vi "TCC.vi"() -> (2 "State out":string="Data: Load Thermal Calibration")   [LabVIEW 2020]
uses:
  DataCluster_TCAL.ctl
  <vilib>/vision/Image Controls.llb/IMAQ Image.ctl
  DataCluster.ctl
  <vilib>/userdefined/High Color/IMAQdx.ctl
  <vilib>/Utility/xml.llb/Write to XML File(string).vi
panel:
  out "Pict Ring":i32(ring)
  in  "Done":bool
  out "Step":string="Step: 4\n\nCalculate temperature!"
  in  "Fixpoint Radius":i32=20 min=3 max=20
  in  "Cluster":T1 {"PCR Size" items=["384 (24x16)", "96 (12x8)"]; "Points"."Top Left"."Y" format="%.2f"; "Points"."Top Left"."X" format="%.2f"; "Points"."Top Right"."Y" format="%.2f"; "Points"."Top Right"."X" format="%.2f"; "Points"."Bottom Left"."Y" format="%.2f"; "Points"."Bottom Left"."X" format="%.2f"; "Points"."Bottom Right"."Y" format="%.2f"; "Points"."Bottom Right"."X" format="%.2f"; "Points"."Fixpoint"."Y" format="%.2f"; "Points"."Fixpoint"."X" format="%.2f"}
  in  "Display Mapping":u32(ring)=10 items=["Default"=10, "Most Significant Bits"=11, "Full Dynamic"=12, "Downshift"=13, "Given Range"=14, "90% Dynamic"=15, "Given Percent Range"=16]
  in  "Image":u32(slide) scale=0.0..242.0
  in  "Help":bool
  out "Tutorial":string="Step: 4\n\nCalculate temperature!"
  in  "Show All Points":bool
  in  "Well Radius":u32=50 min=1 max=100
  in  "PCR Size":u16(ring) items=["384 (24x16)", "96 (12x8)"]
  out "Points":T3[](array[typedef])=[{"X"=103.0, "Y"=94.0}, {"X"=158.04349, "Y"=93.521736}, {"X"=213.08696, "Y"=93.04348}, {"X"=268.13043, "Y"=92.565216}, {"X"=323.17392, "Y"=92.08696}, {"X"=378.2174, "Y"=91.608696}, {"X"=433.26086, "Y"=91.13043}, {"X"=488.30435, "Y"=90.652176}, {"X"=543.34784, "Y"=90.17391}, {"X"=598.39136, "Y"=89.69565}, {"X"=653.4348, "Y"=89.21739}, {"X"=708.4783, "Y"=88.73913}, {"X"=763.5217, "Y"=88.26087}, {"X"=818.56525, "Y"=87.78261}, {"X"=873.6087, "Y"=87.30435}, {"X"=928.6522, "Y"=86.82609}, {"X"=983.6957, "Y"=86.347824}, {"X"=1038.7391, "Y"=85.86957}, {"X"=1093.7827, "Y"=85.391304}, {"X"=1148.8262, "Y"=84.91304}, {"X"=1203.8696, "Y"=84.434784}, {"X"=1258.9131, "Y"=83.95652}, {"X"=1313.9565, "Y"=83.478264}, {"X"=1369.0, "Y"=83.0}, {"X"=103.46667, "Y"=149.06667}, {"X"=158.51015, "Y"=148.58841}, {"X"=213.55362, "Y"=148.11014}, {"X"=268.5971, "Y"=147.63188}, {"X"=323.6406, "Y"=147.15363}, {"X"=378.68408, "Y"=146.67535}, {"X"=433.72754, "Y"=146.1971}, {"X"=488.77103, "Y"=145.71884}, {"X"=543.8145, "Y"=145.24057}, {"X"=598.858, "Y"=144.76231}, {"X"=653.9015, "Y"=144.28406}, {"X"=708.94495, "Y"=143.8058}, {"X"=763.9884, "Y"=143.32753}, {"X"=819.0319, "Y"=142.84927}, {"X"=874.0754, "Y"=142.37102}, {"X"=929.1189, "Y"=141.89276}, {"X"=984.16235, "Y"=141.41449}, {"X"=1039.2058, "Y"=140.93623}, {"X"=1094.2493, "Y"=140.45798}, {"X"=1149.2928, "Y"=139.9797}, {"X"=1204.3363, "Y"=139.50145}, {"X"=1259.3798, "Y"=139.0232}, {"X"=1314.4232, "Y"=138.54492}, {"X"=1369.4667, "Y"=138.06667}, {"X"=103.933334, "Y"=204.13333}, {"X"=158.9768, "Y"=203.65506}, {"X"=214.0203, "Y"=203.17682}, {"X"=269.06375, "Y"=202.69855}, {"X"=324.10724, "Y"=202.22029}, {"X"=379.15073, "Y"=201.74203}, {"X"=434.19418, "Y"=201.26376}, {"X"=489.23767, "Y"=200.7855}, {"X"=544.2812, "Y"=200.30725}, {"X"=599.32465, "Y"=199.82898}, {"X"=654.36816, "Y"=199.35072}, {"X"=709.4116, "Y"=198.87247}, {"X"=764.4551, "Y"=198.3942}, {"X"=819.4986, "Y"=197.91594}, {"X"=874.54205, "Y"=197.43768}, {"X"=929.5856, "Y"=196.95941}, {"X"=984.629, "Y"=196.48116}, {"X"=1039.6725, "Y"=196.0029}, {"X"=1094.716, "Y"=195.52463}, {"X"=1149.7595, "Y"=195.04637}, {"X"=1204.803, "Y"=194.56812}, {"X"=1259.8464, "Y"=194.08984}, {"X"=1314.8899, "Y"=193.6116}, {"X"=1369.9333, "Y"=193.13333}, {"X"=104.4, "Y"=259.2}, {"X"=159.44348, "Y"=258.72174}, {"X"=214.48695, "Y"=258.24347}, {"X"=269.53043, "Y"=257.7652}, {"X"=324.5739, "Y"=257.28696}, {"X"=379.6174, "Y"=256.8087}, {"X"=434.66086, "Y"=256.33044}, {"X"=489.70435, "Y"=255.85217}, {"X"=544.74786, "Y"=255.37392}, {"X"=599.7913, "Y"=254.89565}, {"X"=654.83484, "Y"=254.41739}, {"X"=709.8783, "Y"=253.93913}, {"X"=764.92175, "Y"=253.46086}, {"X"=819.9653, "Y"=252.9826}, {"X"=875.0087, "Y"=252.50435}, {"X"=930.05225, "Y"=252.02608}, {"X"=985.0957, "Y"=251.54782}, {"X"=1040.1392, "Y"=251.06956}, {"X"=1095.1826, "Y"=250.59131}, {"X"=1150.2262, "Y"=250.11304}, {"X"=1205.2697, "Y"=249.63478}, {"X"=1260.3131, "Y"=249.15652}, {"X"=1315.3566, "Y"=248.67825}, {"X"=1370.4, "Y"=248.2}, {"X"=104.86667, "Y"=314.26666}, {"X"=159.91014, "Y"=313.7884}, {"X"=214.95363, "Y"=313.31012}, {"X"=269.9971, "Y"=312.83188}, {"X"=325.0406, "Y"=312.35364}, {"X"=380.08408, "Y"=311.87537}, {"X"=435.12753, "Y"=311.3971}, {"X"=490.17102, "Y"=310.91882}, {"X"=545.2145, "Y"=310.44058}, {"X"=600.258, "Y"=309.9623}, {"X"=655.30145, "Y"=309.48407}, {"X"=710.3449, "Y"=309.0058}, {"X"=765.38837, "Y"=308.52753}, {"X"=820.4319, "Y"=308.04926}, {"X"=875.47534, "Y"=307.571}, {"X"=930.51886, "Y"=307.09274}, {"X"=985.5623, "Y"=306.6145}, {"X"=1040.6058, "Y"=306.13623}, {"X"=1095.6493, "Y"=305.65796}, {"X"=1150.6929, "Y"=305.1797}, {"X"=1205.7363, "Y"=304.70145}, {"X"=1260.7798, "Y"=304.2232}, {"X"=1315.8232, "Y"=303.74493}, {"X"=1370.8667, "Y"=303.26666}, {"X"=105.333336, "Y"=369.3333}, {"X"=160.37682, "Y"=368.85504}, {"X"=215.42029, "Y"=368.3768}, {"X"=270.46378, "Y"=367.89853}, {"X"=325.50726, "Y"=367.42026}, {"X"=380.55075, "Y"=366.94202}, {"X"=435.5942, "Y"=366.46375}, {"X"=490.6377, "Y"=365.98547}, {"X"=545.68115, "Y"=365.50723}, {"X"=600.7247, "Y"=365.02896}, {"X"=655.7681, "Y"=364.5507}, {"X"=710.8116, "Y"=364.07245}, {"X"=765.85504, "Y"=363.59418}, {"X"=820.89856, "Y"=363.11594}, {"X"=875.942, "Y"=362.63766}, {"X"=930.98553, "Y"=362.1594}, {"X"=986.029, "Y"=361.68115}, {"X"=1041.0725, "Y"=361.20288}, {"X"=1096.116, "Y"=360.7246}, {"X"=1151.1595, "Y"=360.24637}, {"X"=1206.203, "Y"=359.7681}, {"X"=1261.2465, "Y"=359.28983}, {"X"=1316.2899, "Y"=358.81158}, {"X"=1371.3334, "Y"=358.3333}, {"X"=105.8, "Y"=424.4}, {"X"=160.84348, "Y"=423.92172}, {"X"=215.88696, "Y"=423.44348}, {"X"=270.93042, "Y"=422.9652}, {"X"=325.9739, "Y"=422.48694}, {"X"=381.0174, "Y"=422.0087}, {"X"=436.06085, "Y"=421.53043}, {"X"=491.10434, "Y"=421.05215}, {"X"=546.1478, "Y"=420.5739}, {"X"=601.19135, "Y"=420.09564}, {"X"=656.2348, "Y"=419.61737}, {"X"=711.27826, "Y"=419.13913}, {"X"=766.3217, "Y"=418.66086}, {"X"=821.36523, "Y"=418.18262}, {"X"=876.4087, "Y"=417.70435}, {"X"=931.4522, "Y"=417.22607}, {"X"=986.49567, "Y"=416.74783}, {"X"=1041.5392, "Y"=416.26956}, {"X"=1096.5826, "Y"=415.7913}, {"X"=1151.6262, "Y"=415.31305}, {"X"=1206.6697, "Y"=414.83478}, {"X"=1261.7131, "Y"=414.3565}, {"X"=1316.7566, "Y"=413.87827}, {"X"=1371.8, "Y"=413.4}, {"X"=106.26667, "Y"=479.46667}, {"X"=161.31015, "Y"=478.9884}, {"X"=216.35362, "Y"=478.51016}, {"X"=271.3971, "Y"=478.0319}, {"X"=326.44058, "Y"=477.55362}, {"X"=381.48407, "Y"=477.07538}, {"X"=436.52753, "Y"=476.5971}, {"X"=491.571, "Y"=476.11884}, {"X"=546.6145, "Y"=475.6406}, {"X"=601.658, "Y"=475.16232}, {"X"=656.7015, "Y"=474.68405}, {"X"=711.74493, "Y"=474.2058}, {"X"=766.7884, "Y"=473.72754}, {"X"=821.8319, "Y"=473.2493}, {"X"=876.87537, "Y"=472.77103}, {"X"=931.9189, "Y"=472.29276}, {"X"=986.96234, "Y"=471.8145}, {"X"=1042.0059, "Y"=471.33624}, {"X"=1097.0493, "Y"=470.85797}, {"X"=1152.0929, "Y"=470.37973}, {"X"=1207.1364, "Y"=469.90146}, {"X"=1262.1798, "Y"=469.4232}, {"X"=1317.2233, "Y"=468.94495}, {"X"=1372.2667, "Y"=468.46667}, {"X"=106.73333, "Y"=534.5333}, {"X"=161.77681, "Y"=534.05505}, {"X"=216.8203, "Y"=533.5768}, {"X"=271.86377, "Y"=533.0985}, {"X"=326.90726, "Y"=532.62024}, {"X"=381.95074, "Y"=532.142}, {"X"=436.9942, "Y"=531.66376}, {"X"=492.0377, "Y"=531.1855}, {"X"=547.0812, "Y"=530.7073}, {"X"=602.12463, "Y"=530.229}, {"X"=657.16815, "Y"=529.75073}, {"X"=712.2116, "Y"=529.27246}, {"X"=767.25507, "Y"=528.7942}, {"X"=822.2986, "Y"=528.3159}, {"X"=877.34204, "Y"=527.83765}, {"X"=932.38556, "Y"=527.3594}, {"X"=987.429, "Y"=526.88116}, {"X"=1042.4724, "Y"=526.4029}, {"X"=1097.516, "Y"=525.9246}, {"X"=1152.5594, "Y"=525.4464}, {"X"=1207.6029, "Y"=524.96814}, {"X"=1262.6464, "Y"=524.48987}, {"X"=1317.6898, "Y"=524.0116}, {"X"=1372.7333, "Y"=523.5333}, {"X"=107.2, "Y"=589.6}, {"X"=162.24348, "Y"=589.1217}, {"X"=217.28696, "Y"=588.64343}, {"X"=272.33044, "Y"=588.16516}, {"X"=327.37393, "Y"=587.6869}, {"X"=382.41742, "Y"=587.2087}, {"X"=437.46088, "Y"=586.7304}, {"X"=492.50436, "Y"=586.25214}, {"X"=547.54785, "Y"=585.7739}, {"X"=602.5913, "Y"=585.29565}, {"X"=657.6348, "Y"=584.8174}, {"X"=712.6783, "Y"=584.3391}, {"X"=767.72174, "Y"=583.86084}, {"X"=822.76526, "Y"=583.38257}, {"X"=877.8087, "Y"=582.9043}, {"X"=932.85223, "Y"=582.426}, {"X"=987.8957, "Y"=581.9478}, {"X"=1042.9391, "Y"=581.46954}, {"X"=1097.9827, "Y"=580.9913}, {"X"=1153.0261, "Y"=580.51306}, {"X"=1208.0696, "Y"=580.0348}, {"X"=1263.113, "Y"=579.5565}, {"X"=1318.1565, "Y"=579.07825}, {"X"=1373.2, "Y"=578.6}, {"X"=107.666664, "Y"=644.6666}, {"X"=162.71014, "Y"=644.18835}, {"X"=217.75363, "Y"=643.7101}, {"X"=272.7971, "Y"=643.2319}, {"X"=327.84058, "Y"=642.7536}, {"X"=382.88406, "Y"=642.2753}, {"X"=437.92752, "Y"=641.79706}, {"X"=492.971, "Y"=641.3188}, {"X"=548.0145, "Y"=640.8405}, {"X"=603.058, "Y"=640.3623}, {"X"=658.1015, "Y"=639.88403}, {"X"=713.14496, "Y"=639.40576}, {"X"=768.1884, "Y"=638.9275}, {"X"=823.23193, "Y"=638.4492}, {"X"=878.2754, "Y"=637.97095}, {"X"=933.3189, "Y"=637.49274}, {"X"=988.36237, "Y"=637.01447}, {"X"=1043.4058, "Y"=636.5362}, {"X"=1098.4493, "Y"=636.0579}, {"X"=1153.4928, "Y"=635.57965}, {"X"=1208.5363, "Y"=635.1014}, {"X"=1263.5797, "Y"=634.62317}, {"X"=1318.6232, "Y"=634.1449}, {"X"=1373.6666, "Y"=633.6666}, {"X"=108.13333, "Y"=699.73334}, {"X"=163.17682, "Y"=699.25507}, {"X"=218.22029, "Y"=698.7768}, {"X"=273.26376, "Y"=698.2986}, {"X"=328.30725, "Y"=697.8203}, {"X"=383.35074, "Y"=697.34204}, {"X"=438.3942, "Y"=696.8638}, {"X"=493.43768, "Y"=696.3855}, {"X"=548.4812, "Y"=695.9072}, {"X"=603.52466, "Y"=695.429}, {"X"=658.5682, "Y"=694.95074}, {"X"=713.61163, "Y"=694.4725}, {"X"=768.6551, "Y"=693.9942}, {"X"=823.6986, "Y"=693.5159}, {"X"=878.74207, "Y"=693.03766}, {"X"=933.7856, "Y"=692.55945}, {"X"=988.82904, "Y"=692.0812}, {"X"=1043.8724, "Y"=691.6029}, {"X"=1098.916, "Y"=691.12463}, {"X"=1153.9595, "Y"=690.64636}, {"X"=1209.0029, "Y"=690.1681}, {"X"=1264.0464, "Y"=689.6899}, {"X"=1319.0898, "Y"=689.2116}, {"X"=1374.1333, "Y"=688.73334}, {"X"=108.6, "Y"=754.8}, {"X"=163.64348, "Y"=754.3217}, {"X"=218.68697, "Y"=753.84344}, {"X"=273.73044, "Y"=753.36523}, {"X"=328.77393, "Y"=752.88696}, {"X"=383.8174, "Y"=752.4087}, {"X"=438.86087, "Y"=751.9304}, {"X"=493.90436, "Y"=751.45215}, {"X"=548.9478, "Y"=750.9739}, {"X"=603.99133, "Y"=750.49567}, {"X"=659.0348, "Y"=750.0174}, {"X"=714.07825, "Y"=749.5391}, {"X"=769.1217, "Y"=749.06085}, {"X"=824.1652, "Y"=748.5826}, {"X"=879.2087, "Y"=748.1043}, {"X"=934.2522, "Y"=747.6261}, {"X"=989.29565, "Y"=747.1478}, {"X"=1044.3391, "Y"=746.66956}, {"X"=1099.3827, "Y"=746.1913}, {"X"=1154.4261, "Y"=745.713}, {"X"=1209.4696, "Y"=745.23474}, {"X"=1264.5131, "Y"=744.75653}, {"X"=1319.5565, "Y"=744.27826}, {"X"=1374.6, "Y"=743.8}, {"X"=109.066666, "Y"=809.86664}, {"X"=164.11015, "Y"=809.38837}, {"X"=219.15363, "Y"=808.9101}, {"X"=274.1971, "Y"=808.4319}, {"X"=329.2406, "Y"=807.9536}, {"X"=384.2841, "Y"=807.47534}, {"X"=439.32755, "Y"=806.9971}, {"X"=494.37103, "Y"=806.5188}, {"X"=549.4145, "Y"=806.0405}, {"X"=604.458, "Y"=805.5623}, {"X"=659.50146, "Y"=805.08405}, {"X"=714.5449, "Y"=804.6058}, {"X"=769.5884, "Y"=804.1275}, {"X"=824.6319, "Y"=803.64923}, {"X"=879.67535, "Y"=803.17096}, {"X"=934.7189, "Y"=802.69275}, {"X"=989.7623, "Y"=802.2145}, {"X"=1044.8058, "Y"=801.7362}, {"X"=1099.8494, "Y"=801.25793}, {"X"=1154.8928, "Y"=800.77966}, {"X"=1209.9363, "Y"=800.3014}, {"X"=1264.9797, "Y"=799.8232}, {"X"=1320.0232, "Y"=799.3449}, {"X"=1375.0667, "Y"=798.86664}, {"X"=109.53333, "Y"=864.93335}, {"X"=164.57681, "Y"=864.4551}, {"X"=219.6203, "Y"=863.9768}, {"X"=274.66376, "Y"=863.4986}, {"X"=329.70724, "Y"=863.0203}, {"X"=384.75073, "Y"=862.54205}, {"X"=439.7942, "Y"=862.0638}, {"X"=494.83768, "Y"=861.5855}, {"X"=549.88116, "Y"=861.10724}, {"X"=604.9247, "Y"=860.629}, {"X"=659.96814, "Y"=860.15076}, {"X"=715.0116, "Y"=859.6725}, {"X"=770.05505, "Y"=859.1942}, {"X"=825.0986, "Y"=858.71594}, {"X"=880.142, "Y"=858.2377}, {"X"=935.18555, "Y"=857.75946}, {"X"=990.229, "Y"=857.2812}, {"X"=1045.2725, "Y"=856.8029}, {"X"=1100.316, "Y"=856.32465}, {"X"=1155.3595, "Y"=855.8464}, {"X"=1210.403, "Y"=855.3681}, {"X"=1265.4464, "Y"=854.8899}, {"X"=1320.4899, "Y"=854.4116}, {"X"=1375.5333, "Y"=853.93335}, {"X"=110.0, "Y"=920.0}, {"X"=165.04349, "Y"=919.5217}, {"X"=220.08696, "Y"=919.04346}, {"X"=275.13043, "Y"=918.56525}, {"X"=330.17392, "Y"=918.087}, {"X"=385.2174, "Y"=917.6087}, {"X"=440.26086, "Y"=917.13043}, {"X"=495.30435, "Y"=916.65216}, {"X"=550.34784, "Y"=916.1739}, {"X"=605.39136, "Y"=915.6957}, {"X"=660.4348, "Y"=915.2174}, {"X"=715.4783, "Y"=914.73914}, {"X"=770.5217, "Y"=914.26086}, {"X"=825.56525, "Y"=913.7826}, {"X"=880.6087, "Y"=913.3043}, {"X"=935.6522, "Y"=912.8261}, {"X"=990.6957, "Y"=912.34784}, {"X"=1045.7391, "Y"=911.86957}, {"X"=1100.7827, "Y"=911.3913}, {"X"=1155.8262, "Y"=910.913}, {"X"=1210.8696, "Y"=910.43475}, {"X"=1265.9131, "Y"=909.95654}, {"X"=1320.9565, "Y"=909.4783}, {"X"=1376.0, "Y"=909.0}] {"Y" format="%.2f"; "X" format="%.2f"}
  out "State":i32=3
  in  "Previous":bool
  in  "Next":bool
  out "Path":path caption="Image Path"
  out "Image":T2(plugin-control)
  # "hints \nPress F1 or F2 to cycle through the steps\nUse the Mouse Wheel to zoom in and out"
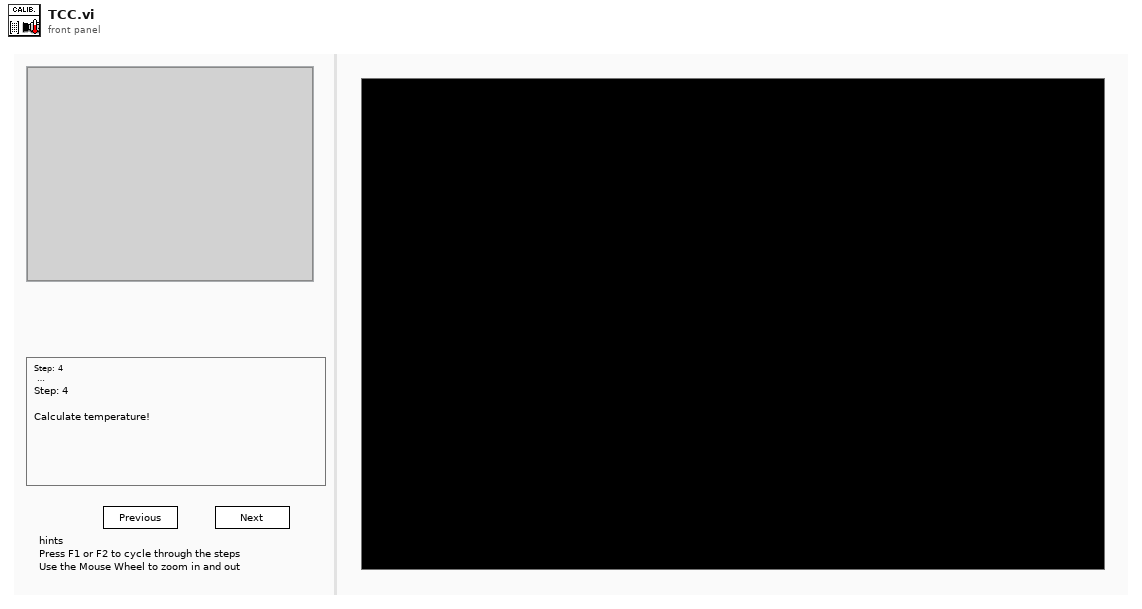
[diagram p1: front panel]
types:
  T1 = typedef "DataCluster_TCAL.ctl" = cluster{"Core":cluster{"Current VI Reference":refnum<vi>, "Close Panel on Exit?":bool}, "Image Out":T2, "State":i32, "Points":cluster{"Top Left":T3, "Top Right":T3, "Bottom Left":T3, "Bottom Right":T3, "x space 2":dbl, "y space 2":sgl, "x_space":sgl, "y_space":sgl, "Pixels":cluster{"X":i32, "Y":i32}[][], "Fixpoint":T3}, "img_array":T2[], "Temps":dbl[], "Temps_Array":dbl[][], "Scan Area":dbl, "Fixpoint Area":dbl, "PCR Size":u16}
  T2 = typedef "IMAQ Image.ctl" = refnum<image>
  T3 = typedef "IMAQ Point" = cluster{"X":sgl, "Y":sgl}
  T4 = enum32{"Invalid", "Standard", "Closed", "Hidden", "Minimized", "Maximized"}
  T5 = enum32{"invalid app kind", "Development System", "Run Time System", "Student Edition", "Embedded LabVIEW", "Evaluation", "Custom"}
  T6 = cluster{"Global Rectangle":i32[], "Contours":cluster{"Contour Type":u32, "ROI Type":u32, "Points":i32[]}[]}
  T7 = typedef "DataCluster.ctl" = cluster{"Core":cluster{"Current VI Reference":refnum<vi>, "Close Panel on Exit?":bool, "Exit":bool, "Initialized?":bool}, "Connections":cluster{"cDAQ":cluster{"Task":refnum<k21>, "Connected":bool, "Active":bool, "ID":string}, "Camera":cluster{"Session":T8, "Connected":bool, "Active":bool, "Placeholder":T2}, "PSU":cluster{"Port":refnum<visa-resource-name>, "Connected":bool, "Active":bool}, "Arduino":cluster{"Port":refnum<visa-resource-name>, "Connected":bool, "Active":bool}}, "Data Acquisition":cluster{"Setup":cluster{"Label":string, "Operator":string, "Notes":string, "TempGrad":dbl, "TargetTemp":dbl, "Sample Volume":dbl}, "Camera":cluster{"Image":T2, "Save Image":T2, "Image Frequency":i32, "Rectangle":T9, "Calibration":cluster{"Top Left":T3, "Top Right":T3, "Bottom Left":T3, "Bottom Right":T3, "Fixpoint":T3, "Scan Area":dbl, "Fixpoint Area":dbl, "Well Pixels":cluster{"X":i32, "Y":i32}[][], "Valid":bool}, "FocusPos":u32, "Display Mapping":u32}, "Thermistor":cluster{"Sample Size":i32, "Calibration":cluster{"B0.100":dbl[], "R25":dbl[], "c":dbl[][], "State":bool[], "V_S":dbl, "R_S":dbl}, "Timing Mode":i32}, "Partition":cluster{"Data":string[][], "Cell Label":string, "Cell Color":u32, "Height":i32, "Width":i32, "Grid":string[][]}, "Queue":cluster{"Size":i32, "Queue":refnum<queue>}, "Sample Rate":i32, "Active":bool, "Ready":bool, "Graph Mode":u16, "Gradient Buffer":i32}, "Control":cluster{"Sample Rate":i32, "PID gains":cluster{"proportional gain (Kc)":dbl, "integral time (Ti, min)":dbl, "derivative time (Td, min)":dbl}}, "Manual Temp Control":cluster{"TargetTemp":dbl, "Mode":u16, "Active":bool}}
  T8 = typedef "IMAQdx.ctl" = refnum<k21>
  T9 = typedef "IMAQ Rectangle" = cluster{"Left":i32, "Top":i32, "Right":i32, "Bottom":i32, "Rotation":dbl}
  T10 = enum16{"open", "replace", "create", "open or create", "replace or create", "replace or create with confirmation"}
  T11 = typedef "ROI Descriptor" = cluster{"Global Rectangle":i32[], "Contours":cluster{"ID":enum32{"External", "Internal"}, "Type":u32, "Coordinates":i32[]}[]}
  T12 = typedef "Image Type" = u32
  T13 = cluster{"Current VI Reference":refnum<vi>, "Close Panel on Exit?":bool}
  T14 = cluster{"Top Left":T3, "Top Right":T3, "Bottom Left":T3, "Bottom Right":T3, "x space 2":dbl, "y space 2":sgl, "x_space":sgl, "y_space":sgl, "Pixels":cluster{"X":i32, "Y":i32}[][], "Fixpoint":T3}
  T15 = cluster{"Top Left":T3, "Top Right":T3, "Bottom Left":T3, "Bottom Right":T3, "Fixpoint":T3, "Scan Area":dbl, "Fixpoint Area":dbl, "Well Pixels":cluster{"X":i32, "Y":i32}[][], "Valid":bool}
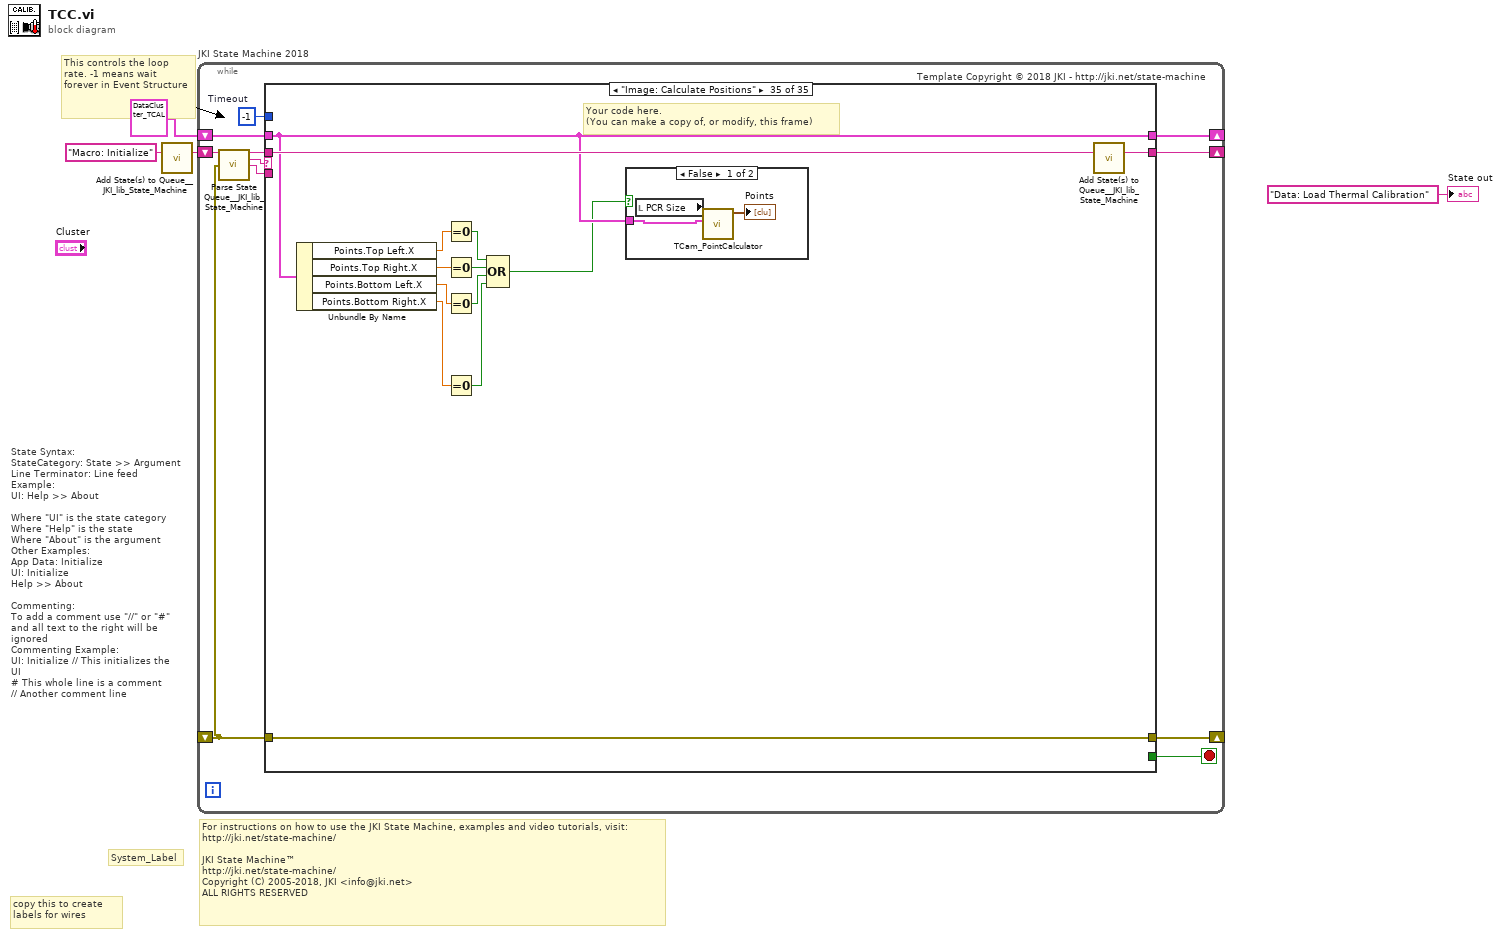
[diagram p0: block diagram]
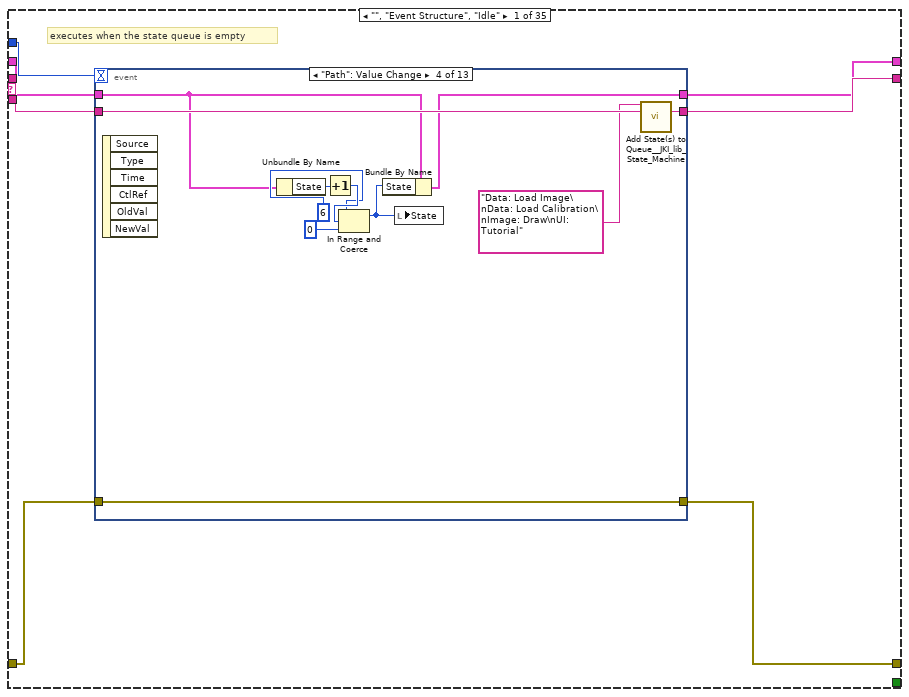
[diagram p2: hidden frame]
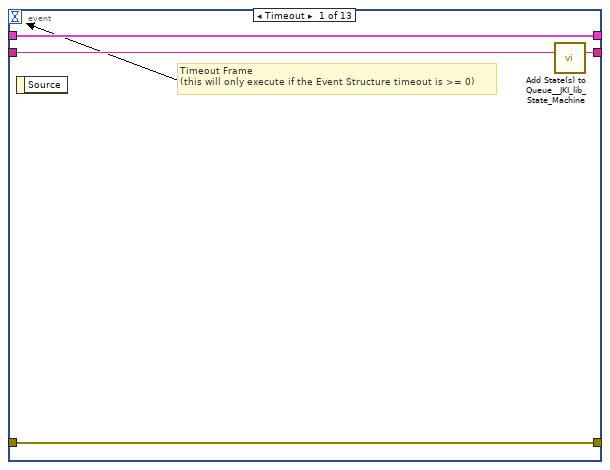
[diagram p3: hidden frame]
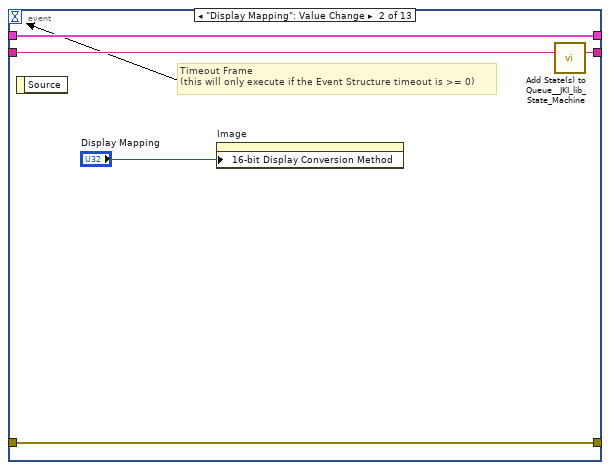
[diagram p4: hidden frame]
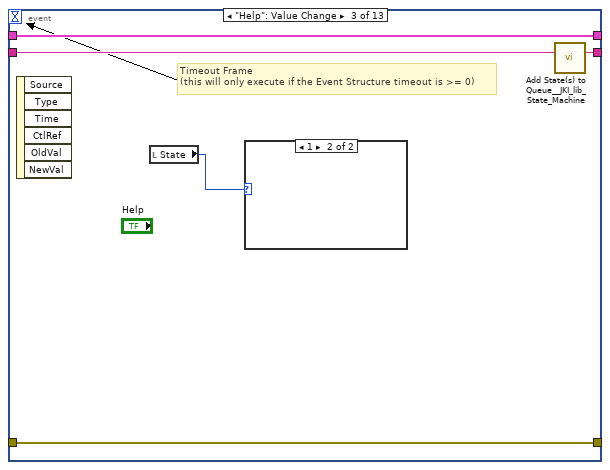
[diagram p5: hidden frame]
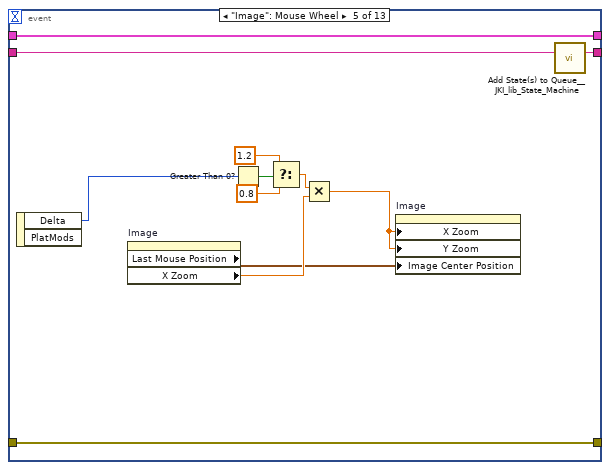
[diagram p7: hidden frame]
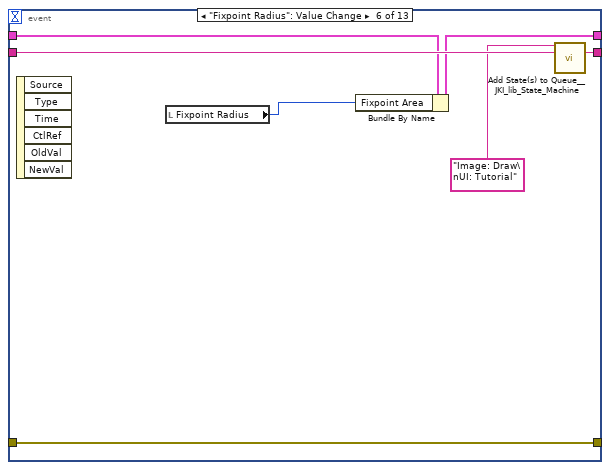
[diagram p8: hidden frame]
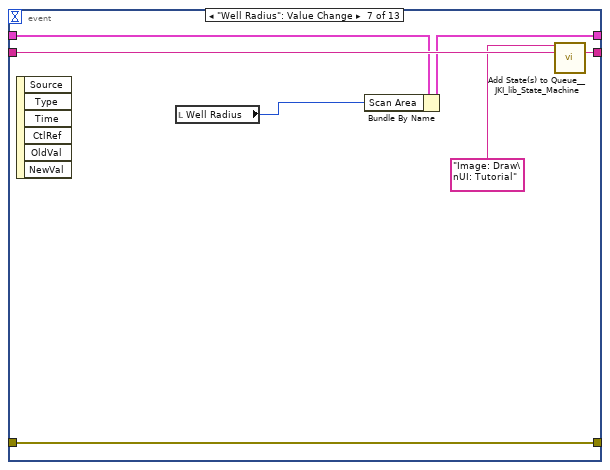
[diagram p9: hidden frame]
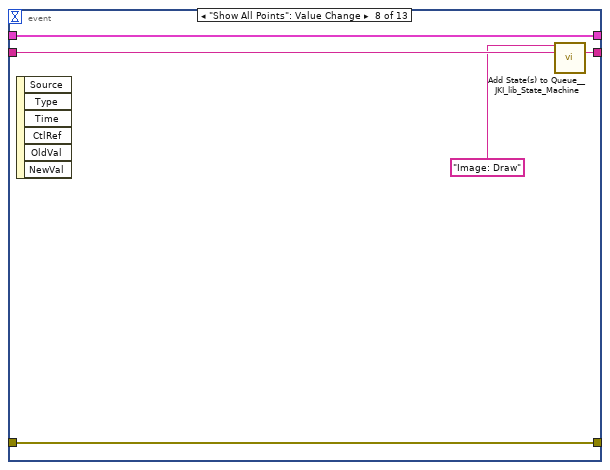
[diagram p10: hidden frame]
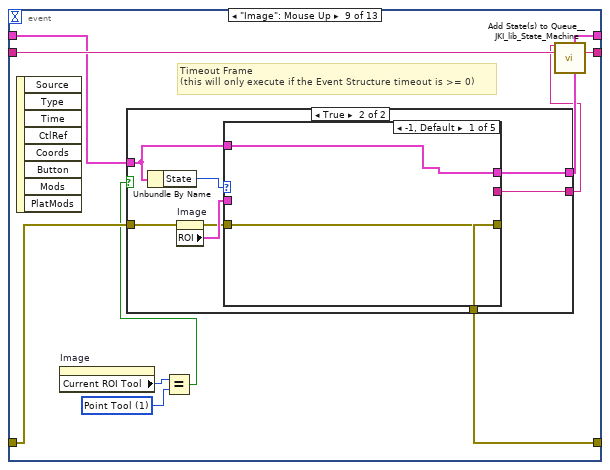
[diagram p11: hidden frame]
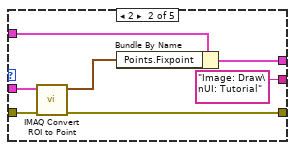
[diagram p13: hidden frame]
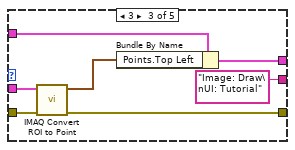
[diagram p14: hidden frame]
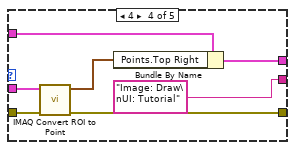
[diagram p15: hidden frame]
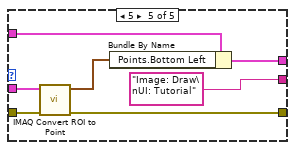
[diagram p16: hidden frame]
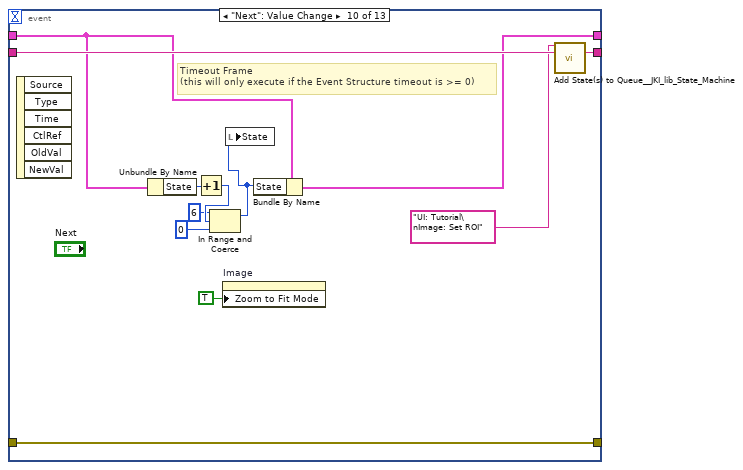
[diagram p17: hidden frame]
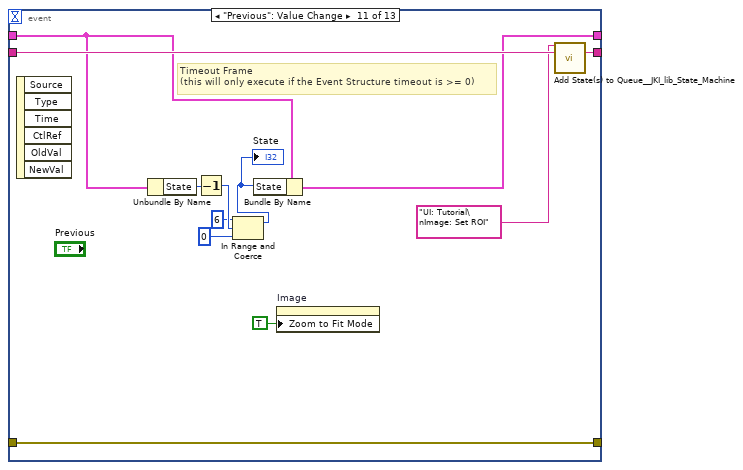
[diagram p18: hidden frame]
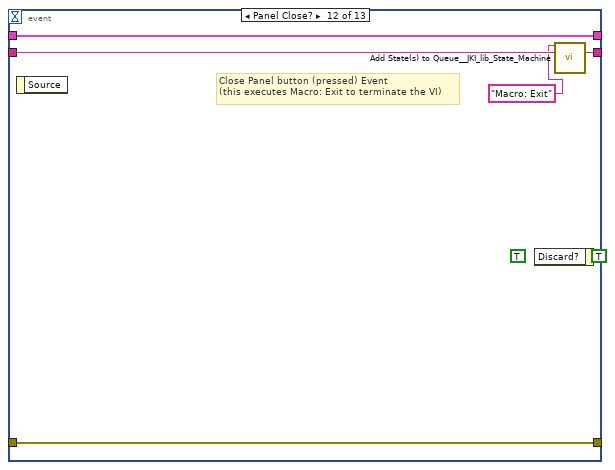
[diagram p19: hidden frame]
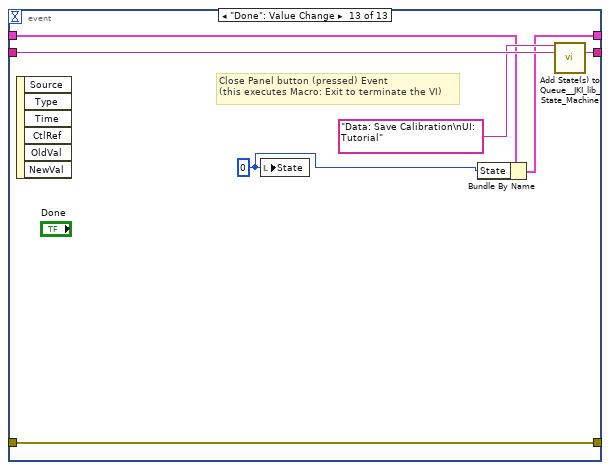
[diagram p20: hidden frame]
diagram:
  # "For instructions on how to use the JKI State Machine, examples and video tutorials, visit:\nhttp://jki.net/state-machine/\n\nJKI State Machine™\nhttp://jki.net/state-machine/\nCopyright (C) 2005-2018, JKI <info@jki.net>\nALL RIGHTS RESERVED"
  # "State Syntax:\nStateCategory: State >> Argument\nLine Terminator: Line feed\nExample:\nUI: Help >> About\n\nWhere \"UI\" is the state category\nWhere \"Help\" is the state\nWhere \"About\" is the argument\nOther Examples:\nApp Data: Initialize\nUI: Initialize\nHelp >> About\n\nCommenting:\nTo add a comment use \"//\" or \"#\" and all text to the right will be ignored\nCommenting Example:\nUI: Initialize // This initializes the UI\n# This whole line is a comment\n// Another comment line"
  # "copy this to create labels for wires"
  # "This controls the loop rate. -1 means wait forever in Event Structure"
  # "System_Label"
  n1 = call <vilib>:"Add State(s) to Queue__JKI_lib_State_Machine.vi"("State(s) in (\"\")"="Macro: Initialize") -> ("States Out"=w4:string)  [unwired: 14 in]
  n2 = while "JKI State Machine 2018" {
    shift-right: [w8] -> _
    shift-left: T1 {"Core"={"Current VI Reference"=refnum, "Close Panel on Exit?"=FALSE}, "Image Out"=refnum, "State"=0, "Points"={"Top Left"={"X"=0.0, "Y"=0.0}, "Top Right"={"X"=0.0, "Y"=0.0}, "Bottom Left"={"X"=0.0, "Y"=0.0}, "Bottom Right"={"X"=0.0, "Y"=0.0}, "x space 2"=0.0, "y space 2"=0.0, "x_space"=0.0, "y_space"=0.0, "Pixels"=[], "Fixpoint"={"X"=0.0, "Y"=0.0}}, "img_array"=[], "Temps"=[], "Temps_Array"=[], "Scan Area"=0.0, "Fixpoint Area"=0.0, "PCR Size"=0} ("output cluster") -> [w7]
    shift-right: [w11] -> _
    shift-left: _ -> [w5]
    shift-right: [w10] -> _
    shift-left: w4 -> [w12]
    stop <- w9 stop-if-true
    w6 = -1  # Timeout
    # "Template Copyright © 2018 JKI - http://jki.net/state-machine"
    n3 = call <vilib>:"Parse State Queue__JKI_lib_State_Machine.vi"("State Queue"=w12, "Error In (no error)"=w5) -> ("Remaining States"=w14:string, "Current State"=w15:string, "Arguments"=w13:string)  [unwired: 11 in]
    n4 = case shown="\"Image: Calculate Positions\"" w15 {
      selector: w15 -> [_ _ w170 _ _ _ _ _ _ _ _ _ _ _ _ _ _ _ _ _ _ _ _ _ _ _ _ _ _ _ _ _ _ _ _]
      tunnel: w14 -> [w22 w169 w174 w193 w199 w204 w208 w221 w252 w257 w275 w288 w329 w357 w378 w398 w416 w477 w488 w557 w562 w573 w577 w582 w587 w607 w624 w630 w648 w668 w686 w697 w725 w790 w812]
      tunnel: w13 -> [_ _ _ _ _ _ _ _ _ _ _ _ _ _ _ _ _ w472 w482 _ _ _ _ _ _ _ _ _ _ _ _ _ w723 _ _]
      tunnel: w7 -> [w20 w166 w172 w186 w196 w202 w205 w210 w249 w253 _ w284 w326 w355 w375 w396 w403 w475 w484 w554 w559 w570 w574 w579 w584 w588 w622 w628 w639 w659 w677 w695 w721 w777 w801]
      tunnel: [w19 w167 w176 w190 errorcluster {"status"=FALSE, "code"=0, "source"=""} ("error out") w201 w206 w215 w246 w255 w266 w285 w323 w338 w376 w395 w414 w473 w485 w555 w560 w571 w575 w580 w585 w605 w617 w625 w646 w666 w684 w690 w718 w787 w810] -> w11
      tunnel: w5 -> [w18 w167 w175 w190 w195 w201 w206 w218 w246 w255 w267 w286 w322 w354 w376 w395 w414 w474 w486 w555 w560 w571 w575 w580 w585 w605 w617 w626 w646 w666 w684 w694 w719 w787 w810]
      tunnel: [w21 w168 w173 w192 w198 w203 w207 w220 w251 w256 w274 w287 w328 w356 w377 w397 w415 w476 w487 w556 w561 w572 w576 w581 w586 w606 w623 w629 w647 w667 w685 w696 w724 w789 w811] -> w10
      tunnel: [_ _ _ _ _ TRUE _ _ _ _ _ _ _ _ _ _ _ _ _ _ _ _ _ _ _ _ _ _ _ _ _ _ _ _ _] -> w9
      tunnel: [w17 w166 w172 w191 w196 w202 w205 w219 w250 w253 w273 w280 w326 w355 w375 w396 w403 w475 w484 w554 w559 w570 w574 w579 w584 w588 w622 w628 w638 w658 w676 w695 w721 w776 w801] -> w8
      tunnel: w6 -> [w16 _ _ _ _ _ _ _ _ _ _ _ _ _ _ _ _ _ _ _ _ _ _ _ _ _ _ _ _ _ _ _ _ _ _]
      frame "", "Event Structure", "Idle" {
        # "executes when the state queue is empty"
        n5 = event shown="[3] \"Path\": Value Change" {
          selector: _ -> [_ _ _ _ _ _ _ _ _ _ _ _ _]
          dyn-events: _ -> [_ _ _ _ _ _ _ _ _ _ _ _ _]
          timeout: w16 -> [_ _ _ _ _ _ _ _ _ _ _ _ _]
          tunnel: w22 -> [w26 w31 w36 w47 w59 w66 w73 w78 w88 w140 w152 w158 w165]
          tunnel: [w25 w30 w35 w46 w58 w65 w72 w77 w87 w139 w151 w157 w164] -> w21
          tunnel: w20 -> [w23 w28 w33 w38 w56 w63 w70 w75 w85 w138 w150 w155 w161]
          tunnel: [w24 w29 w34 w45 w57 w64 w71 w76 w83 w135 w147 w156 w163] -> w19
          tunnel: w18 -> [w24 w29 w34 w45 w57 w64 w71 w76 w86 w135 w147 w156 w163]
          tunnel: [w23 w28 w33 w39 w56 w61 w68 w75 w84 w136 w148 w155 w159] -> w17
          event Timeout {
            # "Timeout Frame\n(this will only execute if the Event Structure timeout is >= 0)"
            n6 = event-data() -> ()  [unwired: 1 in, 1 out]
            n7 = call <vilib>:"Add State(s) to Queue__JKI_lib_State_Machine.vi"("State(s) in (\"\")"=w26) -> ("States Out"=w25:string)  [unwired: 14 in]
          }
          event "Display Mapping": Value Change {
            # "Timeout Frame\n(this will only execute if the Event Structure timeout is >= 0)"
            n8 = event-data() -> ()  [unwired: 1 in, 1 out]
            n9 = property on="Image" class="ImageControl"("16-bit Display Conversion Method"="Display Mapping") -> ()  [unwired: 2 in, 2 out]
            n10 = call <vilib>:"Add State(s) to Queue__JKI_lib_State_Machine.vi"("State(s) in (\"\")"=w31) -> ("States Out"=w30:string)  [unwired: 14 in]
          }
          event "Help": Value Change {
            # "Timeout Frame\n(this will only execute if the Event Structure timeout is >= 0)"
            n11 = event-data() -> ()  [unwired: 1 in, 6 out]
            n12 = local read "State"() -> (w32:i32)
            n13 = case shown="1" w32 {
              frame 0, Default {
              }
              frame 1 {
              }
            }
            n14 = call <vilib>:"Add State(s) to Queue__JKI_lib_State_Machine.vi"("State(s) in (\"\")"=w36) -> ("States Out"=w35:string)  [unwired: 14 in]
          }
          event "Path": Value Change {
            n15 = event-data() -> ()  [unwired: 1 in, 6 out]
            n16 = Unbundle By Name(w38) -> ("State"=w43:i32)
            n17 = Increment(x=w43) -> (x+1=w42:i32)
            n18 = In Range and Coerce(upper limit=6, x=w42, lower limit=0) -> (coerced(x)=w37:i32)  [unwired: 1 out]
            n19 = Bundle By Name(cluster=w38, "State"=w37) -> (w39:T1)
            n20 = local write "State"(w37) -> ()
            n21 = call <vilib>:"Add State(s) to Queue__JKI_lib_State_Machine.vi"("State(s) in Front (\"\")"="Data: Load Image\nData: Load Calibration\nImage: Draw\nUI: Tutorial" ("State(s) in Front (\"\")"), "State(s) in (\"\")"=w47) -> ("States Out"=w46:string)  [unwired: 13 in]
          }
          event "Image": Mouse Wheel {
            n22 = event-data() -> ("Delta"=w55:i32)  [unwired: 1 in, 1 out]
            n23 = property on="Image" class="ImageControl"() -> ("Last Mouse Position"=w49:cluster{"X":i32, "Y":i32}, "X Zoom"=w50:sgl)  [unwired: 2 in, 2 out]
            n24 = Greater Than 0?(x=w55) -> (x > 0?=w54:bool)
            n25 = Select(t=1.2, s=w54, f=0.8) -> (s? t:f=w51:dbl)
            n26 = Multiply(x=w51, y=w50) -> (x*y=w48:dbl)
            n27 = property on="Image" class="ImageControl"("X Zoom"=w48, "Y Zoom"=w48, "Image Center Position"=w49) -> ()  [unwired: 2 in, 2 out]
            n28 = call <vilib>:"Add State(s) to Queue__JKI_lib_State_Machine.vi"("State(s) in (\"\")"=w59) -> ("States Out"=w58:string)  [unwired: 14 in]
          }
          event "Fixpoint Radius": Value Change {
            n29 = event-data() -> ()  [unwired: 1 in, 6 out]
            n30 = local read "Fixpoint Radius"() -> (w60:i32)
            n31 = Bundle By Name(cluster=w63, "Fixpoint Area"=w60) -> (w61:T1)
            n32 = call <vilib>:"Add State(s) to Queue__JKI_lib_State_Machine.vi"("State(s) in Front (\"\")"="Image: Draw\nUI: Tutorial" ("State(s) in Front (\"\")"), "State(s) in (\"\")"=w66) -> ("States Out"=w65:string)  [unwired: 13 in]
          }
          event "Well Radius": Value Change {
            n33 = event-data() -> ()  [unwired: 1 in, 6 out]
            n34 = local read "Well Radius"() -> (w67:u32)
            n35 = Bundle By Name(cluster=w70, "Scan Area"=w67) -> (w68:T1)
            n36 = call <vilib>:"Add State(s) to Queue__JKI_lib_State_Machine.vi"("State(s) in Front (\"\")"="Image: Draw\nUI: Tutorial" ("State(s) in Front (\"\")"), "State(s) in (\"\")"=w73) -> ("States Out"=w72:string)  [unwired: 13 in]
          }
          event "Show All Points": Value Change {
            n37 = event-data() -> ()  [unwired: 1 in, 6 out]
            n38 = call <vilib>:"Add State(s) to Queue__JKI_lib_State_Machine.vi"("State(s) in Front (\"\")"="Image: Draw" ("State(s) in Front (\"\")"), "State(s) in (\"\")"=w78) -> ("States Out"=w77:string)  [unwired: 13 in]
          }
          event "Image": Mouse Up {
            w81 = u32 1 items=["Zoom Tool"=8, "Selection Tool"=0, "Pan Tool"=9, "Point Tool"=1, "Line Tool"=2, "Rectangle Tool"=3, "Rotated Rectangle Tool"=12, "Polyline Tool"=10, "Polygon Tool"=5, "Freehand Tool"=11, "Closed Freehand Tool"=6, "Ellipse Tool"=4, "Annulus Tool"=7] ("Current ROI Tool")
            # "Timeout Frame\n(this will only execute if the Event Structure timeout is >= 0)"
            n39 = event-data() -> ()  [unwired: 1 in, 8 out]
            n40 = property on="Image" class="ImageControl"() -> ("Current ROI Tool"=w82:u32)  [unwired: 2 in, 2 out]
            n41 = Equal?(x=w82, y=w81) -> (x = y?=w80:bool)
            n42 = case shown="True" w80 {
              tunnel: w86 -> [w90 w95]
              tunnel: w85 -> [w89 w94]
              tunnel: [w89 w93] -> w84
              tunnel: [w90 w92] -> w83
              tunnel: [_ w91] -> w79
              frame False {
              }
              frame True {
                n43 = Unbundle By Name(w94) -> ("State"=w98:i32)
                n44 = property on="Image" class="ImageControl"(error in=w95) -> (error out=w96:errorcluster, "ROI"=w97:T6)  [unwired: 1 in, 1 out]
                n45 = case shown="-1, Default" w98 {
                  tunnel: w97 -> [_ w106 w113 w121 w128]
                  tunnel: w96 -> [w99 w105 w112 w120 w127]
                  tunnel: w94 -> [w100 w102 w109 w119 w126]
                  tunnel: [w100 w103 w110 w118 w125] -> w93
                  tunnel: [w99 w104 w111 w116 w123] -> w92
                  tunnel: [_ "Image: Draw\nUI: Tutorial" "Image: Draw\nUI: Tutorial" "Image: Draw\nUI: Tutorial" "Image: Draw\nUI: Tutorial"] -> w91
                  frame -1, Default {
                  }
                  frame 2 {
                    n46 = call "IMAQ Convert ROI to Point"("error in (no error)"=w105, "ROI Descriptor"=w106) -> ("error out"=w104:errorcluster, "Point"=w107:T3)  [unwired: 7 in]
                    n47 = Bundle By Name(cluster=w102, "Points.Fixpoint"=w107) -> (w103:T1)
                  }
                  frame 3 {
                    n48 = call "IMAQ Convert ROI to Point"("error in (no error)"=w112, "ROI Descriptor"=w113) -> ("error out"=w111:errorcluster, "Point"=w114:T3)  [unwired: 7 in]
                    n49 = Bundle By Name(cluster=w109, "Points.Top Left"=w114) -> (w110:T1)
                  }
                  frame 4 {
                    n50 = call "IMAQ Convert ROI to Point"("error in (no error)"=w120, "ROI Descriptor"=w121) -> ("error out"=w116:errorcluster, "Point"=w117:T3)  [unwired: 7 in]
                    n51 = Bundle By Name(cluster=w119, "Points.Top Right"=w117) -> (w118:T1)
                  }
                  frame 5 {
                    n52 = call "IMAQ Convert ROI to Point"("error in (no error)"=w127, "ROI Descriptor"=w128) -> ("error out"=w123:errorcluster, "Point"=w124:T3)  [unwired: 7 in]
                    n53 = Bundle By Name(cluster=w126, "Points.Bottom Left"=w124) -> (w125:T1)
                  }
                }
              }
            }
            n54 = call <vilib>:"Add State(s) to Queue__JKI_lib_State_Machine.vi"("State(s) in Front (\"\")"=w79, "State(s) in (\"\")"=w88) -> ("States Out"=w87:string)  [unwired: 13 in]
          }
          event "Next": Value Change {
            # "Timeout Frame\n(this will only execute if the Event Structure timeout is >= 0)"
            n55 = event-data() -> ()  [unwired: 1 in, 6 out]
            n56 = Unbundle By Name(w138) -> ("State"=w137:i32)
            n57 = Increment(x=w137) -> (x+1=w133:i32)
            n58 = In Range and Coerce(upper limit=6, x=w133, lower limit=0) -> (coerced(x)=w130:i32)  [unwired: 1 out]
            n59 = property on="Image" class="ImageControl"("Zoom to Fit Mode"=TRUE) -> ()  [unwired: 2 in, 2 out]
            n60 = local write "State"(w130) -> ()
            n61 = Bundle By Name(cluster=w138, "State"=w130) -> (w136:T1)
            n62 = call <vilib>:"Add State(s) to Queue__JKI_lib_State_Machine.vi"("State(s) in Front (\"\")"="UI: Tutorial\nImage: Set ROI" ("f"), "State(s) in (\"\")"=w140) -> ("States Out"=w139:string)  [unwired: 13 in]
          }
          event "Previous": Value Change {
            # "Timeout Frame\n(this will only execute if the Event Structure timeout is >= 0)"
            n63 = event-data() -> ()  [unwired: 1 in, 6 out]
            n64 = Unbundle By Name(w150) -> ("State"=w149:i32)
            n65 = Decrement(x=w149) -> (x-1=w144:i32)
            n66 = In Range and Coerce(upper limit=6, x=w144, lower limit=0) -> (coerced(x)=w145:i32)  [unwired: 1 out]
            "State" <- w145
            n67 = Bundle By Name(cluster=w150, "State"=w145) -> (w148:T1)
            n68 = property on="Image" class="ImageControl"("Zoom to Fit Mode"=TRUE) -> ()  [unwired: 2 in, 2 out]
            n69 = call <vilib>:"Add State(s) to Queue__JKI_lib_State_Machine.vi"("State(s) in Front (\"\")"="UI: Tutorial\nImage: Set ROI" ("f"), "State(s) in (\"\")"=w152) -> ("States Out"=w151:string)  [unwired: 13 in]
          }
          event Panel Close? {
            (unwired) TRUE ("Discard?")
            # "Close Panel button (pressed) Event\n(this executes Macro: Exit to terminate the VI)"
            n70 = event-data() -> ()  [unwired: 1 in, 1 out]
            n71 = event-data("Discard?"=TRUE) -> ()  [unwired: 1 in, 1 out]
            n72 = call <vilib>:"Add State(s) to Queue__JKI_lib_State_Machine.vi"("State(s) in Front (\"\")"="Macro: Exit", "State(s) in (\"\")"=w158) -> ("States Out"=w157:string)  [unwired: 13 in]
          }
          event "Done": Value Change {
            w160 = 0 ("lower limit")
            # "Close Panel button (pressed) Event\n(this executes Macro: Exit to terminate the VI)"
            n73 = event-data() -> ()  [unwired: 1 in, 6 out]
            n74 = local write "State"(w160) -> ()
            n75 = Bundle By Name(cluster=w161, "State"=w160) -> (w159:T1)
            n76 = call <vilib>:"Add State(s) to Queue__JKI_lib_State_Machine.vi"("State(s) in Front (\"\")"="Data: Save Calibration\nUI: Tutorial", "State(s) in (\"\")"=w165) -> ("States Out"=w164:string)  [unwired: 13 in]
          }
        }
      }
      frame "---------- Core ----------" {
        # "Do not put any code in this frame.\n(it is a separator no-op)"
        n77 = call <vilib>:"Add State(s) to Queue__JKI_lib_State_Machine.vi"("State(s) in (\"\")"=w169) -> ("States Out"=w168:string)  [unwired: 14 in]
      }
      frame Default {
        w179 = 42 items=["No error", "Argument error", "Memory is full", "Out of zone", "End of file", "File already open", "Generic file I/O error", "File not found", "File permission error", "Disk is full", "Duplicate path", "Too many files open", "System feature not enabled", "Resource file not found", "Cannot add resource", "Resource not found", "Image not found", "Image memory error", "Pen does not exist", "Config type invalid", "Config token not found", "Config parse error", "Config memory error", "Bad external code format", "Bad external code offset", "External code not present", "Null window", "Destroy window error", "Null menu", "Print aborted", "Bad print record", "Print driver error", "Windows error during printing", "Memory error during printing", "Print dialog error", "Generic print error", "Invalid device refnum", "Device not found", "Device parameter error", "Device unit error", "Cannot open device", "Device call aborted", "Generic error", "Cancelled by user", "Object ID too low", "Object ID too high", "Object not in heap", "Unknown heap", "Unknown object (invalid DefProc)", "Unknown object (DefProc not in table)", "Message out of range", "Invalid (null) method", "Unknown message", "Manager call not supported", "Bad address", "Network operation in progress", "Network operation timed out", "Connection is busy", "Network attribute not supported", "Network error", "Address in use", "System out of memory", "Connection aborted", "Connection refused", "Not connected", "Already connected", "Connection closed", "Initialization error (interapplication manager)", "Bad occurrence", "Wait on unbound occurrence handler", "Occurrence queue overflow", "Datalog type conflict", "Unused", "Unrecognized type (interapplication manager)", "Memory corrupt", "Failed to make temporary DLL", "Old CIN version", "Drag socket not found", "Failed to load drop-object", "Failed to register OLE object", "Failed to release OLE object", "Format specifier type mismatch", "Unknown format specifier", "Too few format specifiers", "Too many format specifiers", "Scan failed", "Newer CIN version", "Error converting to variant", "Runtime menu error", "Password tampered", "Variant attribute not found", "Incompatible variant data type", "Event data is not available", "Event Store is not present", "Occurrence is not found", "Event Queue is not created", "Event info is not available", "Refnum passed is NULL", "Error retrieving Class GUID", "Error retrieving CoClass GUID", "Error retrieving TypeLib GUID.", "Bad built application magic bytes.", "Specific driver is different from the specific driver associated with the Logical Name.", "There is no session opened to the class driver.", "Max Error", "MAX - Error with config objects", "MAX - Error loading configuration", "MAX - Group not supported"]
        # "Current State"
        # "Do not delete, rename, or modify this frame.\n(this is used to capture unhandled states and typos)"
        # "Handle mistyped state name (developer tool)"
        n78 = Format Into String(format string="Software Exception: Unhandled State \"%s\"." ("message"), error in=w175, w170) -> (resulting string=w178:string, error out=w177:errorcluster)  [unwired: 1 in]
        n79 = call <vilib>:"Error Cluster From Error Code.vi"("show call chain? (False)"=TRUE, "error in (no error)"=w177, "error message (\"\")"=w178, "error code (0)"=w179) -> ("error out"=w176:errorcluster)  [unwired: 5 in]
        n80 = call <vilib>:"Add State(s) to Queue__JKI_lib_State_Machine.vi"("State(s) in (\"\")"=w174) -> ("States Out"=w173:string)  [unwired: 14 in]
      }
      frame "Initialize Core Data" {
        # "Do not delete, rename, or modify this frame.\n(this is used to determine panel behavior on exit)"
        # "originally closed?"
        # "exe?"
        # "If panel starts closed or is an EXE, then close it when we exit"
        n81 = property class="App"() -> ("App.Kind"=w189:T5)  [unwired: 2 in, 2 out]
        n82 = control-ref of="Current VI Reference"() -> (w184:refnum<vi>)
        n83 = property class="VI"() -> ("FP.State"=w183:T4)  [unwired: 2 in, 2 out]
        n84 = Equal?(x=w183, y=T4."Closed" ("Front Panel Window:State")) -> (x = y?=w181:bool)
        n85 = Equal?(x=w189, y=T5."Run Time System" ("Application:Kind")) -> (x = y?=w187:bool)
        n86 = Or(x=w181, y=w187) -> (x .or. y?=w185:bool)
        n87 = Bundle By Name(cluster=w186, "Core.Current VI Reference"=w184, "Core.Close Panel on Exit?"=w185) -> (w191:T1)
        n88 = call <vilib>:"Add State(s) to Queue__JKI_lib_State_Machine.vi"("State(s) in (\"\")"=w193) -> ("States Out"=w192:string)  [unwired: 14 in]
      }
      frame "Error Handler" {
        # "Unhandled Error -- Display it"
        # "Handle any errors here.\nYou can also output any states to clean-up after errors occur"
        # "Clear error"
        n89 = call <vilib>:"General Error Handler.vi"("error in (no error)"=w195) -> ()  [unwired: 10 in, 5 out]
        n90 = call <vilib>:"Add State(s) to Queue__JKI_lib_State_Machine.vi"("State(s) in Front (\"\")"="/* Post Error States", "State(s) in (\"\")"=w199) -> ("States Out"=w198:string)  [unwired: 13 in]
      }
      frame "Exit" {
        # "Do not put any code in this frame.\n(No errors that occur here will be handled.)"
        n91 = call <vilib>:"Add State(s) to Queue__JKI_lib_State_Machine.vi"("State(s) in (\"\")"=w204) -> ("States Out"=w203:string)  [unwired: 14 in]
      }
      frame "---------- Data ----------" {
        # "Do not put any code in this frame.\n(It is a separator no-op. You can make a copy of this frame to create a new Data frame)"
        n92 = call <vilib>:"Add State(s) to Queue__JKI_lib_State_Machine.vi"("State(s) in (\"\")"=w208) -> ("States Out"=w207:string)  [unwired: 14 in]
      }
      frame "Data: Load Image" {
        # "Do not put any code in this frame.\n(It is a separator no-op. You can make a copy of this frame to create a new Data frame)"
        n93 = call "CalibrationImageLoadPrompt.vi"() -> ("cancel?"=w212:bool, "selected path"=w214:path)  [unwired: 10 in]
        "Path" <- w214
        n94 = Empty String/Path?(string/path=w214) -> (empty?=w217:bool)
        n95 = Or(x=w217, y=w212) -> (x .or. y?=w213:bool)
        n96 = case shown="True" w213 {
          tunnel: w218 -> [w229 w244]
          tunnel: [w238 w244] -> w215
          tunnel: w214 -> [w237 _]
          tunnel: [w231 _] -> w216
          tunnel: ["Data: Load Calibration\nImage: Draw\nUI: Tutorial" ("State(s) in Front (\"\")") "" ("State(s) in Front (\"\")")] -> w211
          tunnel: w210 -> [w223 w242]
          tunnel: [w222 w241] -> w209
          frame False {
            w233 = T12 7 items=["Grayscale (U8)", "Grayscale (I16)", "Grayscale (SGL)", "Complex (CSG)", "RGB (U32)", "HSL (U32)", "RGB (U64)", "Grayscale (U16)"] ("Image Type")
            n97 = Unbundle By Name(w223) -> ("State"=w227:i32)
            n98 = Increment(x=w227) -> (x+1=w226:i32)
            n99 = call "IMAQ Create"("Image Name"="img_in", "Image Type"=w233, "error in (no error)"=w229) -> ("New Image"=w235:T2, "error out"=w236:errorcluster)  [unwired: 2 in]
            n100 = In Range and Coerce(upper limit=6, x=w226, lower limit=0) -> (coerced(x)=w222:i32)  [unwired: 1 out]
            n101 = call "IMAQ ReadFile 2"("File Path"=w237, "error in (no error)"=w236, "Image"=w235) -> ("error out"=w234:errorcluster, "Image Out"=w232:T2)  [unwired: 4 in, 3 out]
            n102 = local write "State"(w222) -> ()
            n103 = call "IMAQ Clear Overlay"("error in (no error)"=w234, "Image"=w232) -> ("error out"=w240:errorcluster, "Image Out"=w231:T2)  [unwired: 8 in]
            "Image" <- w231
            n104 = property on="Image" class="ImageControl"(error in=w240, "ROI"=T6 {"Global Rectangle"=[], "Contours"=[]}) -> (error out=w238:errorcluster)  [unwired: 1 in, 1 out]
          }
          frame True {
            n105 = Unbundle By Name(w242) -> ("State"=w241:i32)
          }
        }
        n106 = Bundle By Name(cluster=w210, "Image Out"=w216, "State"=w209) -> (w219:T1)
        n107 = call <vilib>:"Add State(s) to Queue__JKI_lib_State_Machine.vi"("State(s) in Front (\"\")"=w211, "State(s) in (\"\")"=w221) -> ("States Out"=w220:string)  [unwired: 13 in]
      }
      frame "Data: Set Image" {
        # "Do not put any code in this frame.\n(It is a separator no-op. You can make a copy of this frame to create a new Data frame)"
        n108 = Unbundle By Name(w249) -> ("img_array"=w248:T2[])
        n109 = Index Array(array=w248, index="Image") -> (element=w245:T2)
        n110 = Bundle By Name(cluster=w249, "Image Out"=w245) -> (w250:T1)
        n111 = call <vilib>:"Add State(s) to Queue__JKI_lib_State_Machine.vi"("State(s) in (\"\")"=w252) -> ("States Out"=w251:string)  [unwired: 14 in]
      }
      frame "Data: Show Img" {
        # "Do not put any code in this frame.\n(It is a separator no-op. You can make a copy of this frame to create a new Data frame)"
        n112 = Unbundle By Name(w253) -> ("Image Out"=w254:T2)
        n113 = local write "Image"(w254) -> ()
        n114 = call <vilib>:"Add State(s) to Queue__JKI_lib_State_Machine.vi"("State(s) in (\"\")"=w257) -> ("States Out"=w256:string)  [unwired: 14 in]
      }
      frame "Data: Initialize" {
        w268 = dbl[][] []  # Temps_Array
        w269 = dbl[] []  # Temps
        w270 = T2[] []  # img_array
        w264 = 0  # State
        w272 = T13 {"Current VI Reference"=refnum, "Close Panel on Exit?"=FALSE}  # Core
        # "Initialize the shift-register data, here.\n(data names are defined by what you wire into the bundle function)"
        n115 = call <vilib>:"Application Directory.vi"() -> ("Application Directory"=w260:path)
        n116 = Build Path(base path=w260, name or relative path=path "TCam.ini") -> (appended path=w258:path)
        n117 = call "TCam_Calibration_LoadSettings.vi"("error in (no error)"=w267, "path"=w258) -> ("error out"=w266:errorcluster, "Fixpoint Area"=w262:dbl, "Scan Area"=w263:dbl, "Points"=w265:T14)  [unwired: 6 in]
        n118 = local write "Fixpoint Radius"(w262) -> ()
        n119 = local write "Well Radius"(w263) -> ()
        n120 = local write "State"(w264) -> ()
        n121 = Bundle(cluster=T1 {"Core"={"Current VI Reference"=refnum, "Close Panel on Exit?"=FALSE}, "Image Out"=refnum, "State"=0, "Points"={"Top Left"={"X"=0.0, "Y"=0.0}, "Top Right"={"X"=0.0, "Y"=0.0}, "Bottom Left"={"X"=0.0, "Y"=0.0}, "Bottom Right"={"X"=0.0, "Y"=0.0}, "x space 2"=0.0, "y space 2"=0.0, "x_space"=0.0, "y_space"=0.0, "Pixels"=[], "Fixpoint"={"X"=0.0, "Y"=0.0}}, "img_array"=[], "Temps"=[], "Temps_Array"=[], "Scan Area"=0.0, "Fixpoint Area"=0.0, "PCR Size"=0} ("output cluster"), "Core"=w272, "Image Out"=T2 refnum, "State"=w264, "Points"=w265, "img_array"=w270, "Temps"=w269, "Temps_Array"=w268) -> (w273:T1)  [unwired: 3 in]
        n122 = call <vilib>:"Add State(s) to Queue__JKI_lib_State_Machine.vi"("State(s) in (\"\")"=w275) -> ("States Out"=w274:string)  [unwired: 14 in]
      }
      frame "Data: Load Calibration" {
        # "Initialize the shift-register data, here.\n(data names are defined by what you wire into the bundle function)"
        n123 = local read "Path"() -> (w283:path)
        n124 = Strip Path(path=w283) -> (stripped path=w277:path)  [unwired: 1 out]
        n125 = Strip Path(path=w277) -> (stripped path=w276:path)  [unwired: 1 out]
        n126 = Build Path(base path=w276, name or relative path=path "TCC.cal") -> (appended path=w281:path)
        n127 = call <vilib>:"Check if File or Folder Exists.vi"("path"=w281) -> ("file or folder exists?"=w279:bool, "dup path"=w278:path)  [unwired: 8 in, 1 out]
        n128 = case shown="True" w279 {
          tunnel: w286 -> [w289 w298]
          tunnel: [w289 w297] -> w285
          tunnel: w284 -> [w290 w294]
          tunnel: [w290 w292] -> w280
          tunnel: w278 -> [_ w291]
          frame False {
          }
          frame True {
            n129 = call "TCam_Calibration_LoadSettings.vi"("error in (no error)"=w298, "path"=w291) -> ("error out"=w297:errorcluster, "Fixpoint Area"=w295:dbl, "Scan Area"=w296:dbl, "Points"=w293:T14)  [unwired: 6 in]
            n130 = local write "Fixpoint Radius"(w295) -> ()
            n131 = local write "Well Radius"(w296) -> ()
            n132 = Bundle By Name(cluster=w294, "Points"=w293) -> (w292:T1)
          }
        }
        n133 = call <vilib>:"Add State(s) to Queue__JKI_lib_State_Machine.vi"("State(s) in (\"\")"=w288) -> ("States Out"=w287:string)  [unwired: 14 in]
      }
      frame "Data: Cleanup" {
        # "Cleanup any data and references, here.\n(this is called automatically, by the Macro: Exit)"
        n134 = Unbundle By Name(w326) -> ("Points.Top Left"=w319:T3, "Points.Top Right"=w318:T3, "Points.Bottom Left"=w317:T3, "Points.Bottom Right"=w316:T3, "Points.Fixpoint"=w312:T3, "Core.Current VI Reference"=w327:refnum<vi>)
        n135 = local read "Fixpoint Radius"() -> (w310:i32)
        n136 = local read "Well Radius"() -> (w315:u32)
        n137 = Unbundle By Name(T7 {"Core"={"Current VI Reference"=refnum, "Close Panel on Exit?"=FALSE, "Exit"=FALSE, "Initialized?"=FALSE}, "Connections"={"cDAQ"={"Task"="", "Connected"=FALSE, "Active"=FALSE, "ID"=""}, "Camera"={"Session"="", "Connected"=FALSE, "Active"=FALSE, "Placeholder"=refnum}, "PSU"={"Port"="", "Connected"=FALSE, "Active"=FALSE}, "Arduino"={"Port"="", "Connected"=FALSE, "Active"=FALSE}}, "Data Acquisition"={"Setup"={"Label"="", "Operator"="", "Notes"="", "TempGrad"=1.0, "TargetTemp"=1.0, "Sample Volume"=1.0}, "Camera"={"Image"=refnum, "Save Image"=refnum, "Image Frequency"=20, "Rectangle"={"Left"=0, "Top"=0, "Right"=0, "Bottom"=0, "Rotation"=0.0}, "Calibration"={"Top Left"={"X"=0.0, "Y"=0.0}, "Top Right"={"X"=0.0, "Y"=0.0}, "Bottom Left"={"X"=0.0, "Y"=0.0}, "Bottom Right"={"X"=0.0, "Y"=0.0}, "Fixpoint"={"X"=0.0, "Y"=0.0}, "Scan Area"=5.0, "Fixpoint Area"=0.0, "Well Pixels"=[], "Valid"=FALSE}, "FocusPos"=0, "Display Mapping"=10}, "Thermistor"={"Sample Size"=1, "Calibration"={"B0.100"=[], "R25"=[], "c"=[], "State"=[], "V_S"=5.0, "R_S"=100.0}, "Timing Mode"=14713}, "Partition"={"Data"=[], "Cell Label"="", "Cell Color"=0, "Height"=10, "Width"=16, "Grid"=[]}, "Queue"={"Size"=1, "Queue"=refnum}, "Sample Rate"=20, "Active"=FALSE, "Ready"=FALSE, "Graph Mode"=0, "Gradient Buffer"=2}, "Control"={"Sample Rate"=1, "PID gains"={"proportional gain (Kc)"=1.0, "integral time (Ti, min)"=0.01, "derivative time (Td, min)"=0.0}}, "Manual Temp Control"={"TargetTemp"=1.0, "Mode"=0, "Active"=FALSE}} ("Default values")) -> ("Data Acquisition.Camera.Calibration"=w308:T15)
        n138 = Bundle(cluster=w308, "Top Left"=w319, "Top Right"=w318, "Bottom Left"=w317, "Bottom Right"=w316, "Fixpoint"=w312, "Scan Area"=w315, "Fixpoint Area"=w310, "Well Pixels"=cluster{"X":i32, "Y":i32}[][] [], "Valid"=FALSE) -> (w320:T15)
        n139 = call <vilib>:"Application Directory.vi"() -> ("Application Directory"=w307:path)
        n140 = Build Path(base path=w307, name or relative path=path "TCam.ini") -> (appended path=w305:path)
        n141 = call <vilib>:"Check if File or Folder Exists.vi"("error in (no error)"=w322, "path"=w305) -> ("error out"=w302:errorcluster, "file or folder exists?"=w304:bool, "dup path"=w303:path)  [unwired: 7 in]
        n142 = case shown="False" w304 {
          tunnel: w303 -> [w330 w334]
          tunnel: w302 -> [w332 w335]
          tunnel: [w331 w335] -> w301
          tunnel: [w330 w334] -> w300
          frame False {
            n143 = Open/Create/Replace File(file path (use dialog)=w330, error in=w332, operation (0:open)=T10."create") -> (error out=w331:errorcluster)  [unwired: 3 in, 2 out]
          }
          frame True {
          }
        }
        n144 = Flatten To XML(6:w320) -> (2:w299:string)
        n145 = call-poly <vilib>:"Write to XML File.vi"("error in (no error)"=w301, "XML Input"=w299, "XML File Path"=w300) -> ("error out"=w321:errorcluster)  [unwired: 6 in, 2 out]
        n146 = local read "Image"() -> (w311:T2)
        n147 = Close Reference(reference=w327, error in (no error)=w321) -> (error out=w324:errorcluster)
        n148 = call "IMAQ Dispose"("All Images? (No)"=FALSE, "Image"=w311, "error in (no error)"=w324) -> ("error out"=w323:errorcluster)  [unwired: 3 in]
        n149 = call <vilib>:"Add State(s) to Queue__JKI_lib_State_Machine.vi"("State(s) in (\"\")"=w329) -> ("States Out"=w328:string)  [unwired: 14 in]
      }
      frame "Data: Save Calibration" {
        # "Cleanup any data and references, here.\n(this is called automatically, by the Macro: Exit)"
        n150 = local read "Fixpoint Radius"() -> (w344:i32)
        n151 = Unbundle By Name(w355) -> ("Points.Top Left"=w352:T3, "Points.Top Right"=w351:T3, "Points.Bottom Left"=w350:T3, "Points.Bottom Right"=w349:T3, "Points.Fixpoint"=w345:T3)
        n152 = local read "Well Radius"() -> (w348:u32)
        n153 = Unbundle By Name(T7 {"Core"={"Current VI Reference"=refnum, "Close Panel on Exit?"=FALSE, "Exit"=FALSE, "Initialized?"=FALSE}, "Connections"={"cDAQ"={"Task"="", "Connected"=FALSE, "Active"=FALSE, "ID"=""}, "Camera"={"Session"="", "Connected"=FALSE, "Active"=FALSE, "Placeholder"=refnum}, "PSU"={"Port"="", "Connected"=FALSE, "Active"=FALSE}, "Arduino"={"Port"="", "Connected"=FALSE, "Active"=FALSE}}, "Data Acquisition"={"Setup"={"Label"="", "Operator"="", "Notes"="", "TempGrad"=1.0, "TargetTemp"=1.0, "Sample Volume"=1.0}, "Camera"={"Image"=refnum, "Save Image"=refnum, "Image Frequency"=20, "Rectangle"={"Left"=0, "Top"=0, "Right"=0, "Bottom"=0, "Rotation"=0.0}, "Calibration"={"Top Left"={"X"=0.0, "Y"=0.0}, "Top Right"={"X"=0.0, "Y"=0.0}, "Bottom Left"={"X"=0.0, "Y"=0.0}, "Bottom Right"={"X"=0.0, "Y"=0.0}, "Fixpoint"={"X"=0.0, "Y"=0.0}, "Scan Area"=5.0, "Fixpoint Area"=0.0, "Well Pixels"=[], "Valid"=FALSE}, "FocusPos"=0, "Display Mapping"=10}, "Thermistor"={"Sample Size"=1, "Calibration"={"B0.100"=[], "R25"=[], "c"=[], "State"=[], "V_S"=5.0, "R_S"=100.0}, "Timing Mode"=14713}, "Partition"={"Data"=[], "Cell Label"="", "Cell Color"=0, "Height"=10, "Width"=16, "Grid"=[]}, "Queue"={"Size"=1, "Queue"=refnum}, "Sample Rate"=20, "Active"=FALSE, "Ready"=FALSE, "Graph Mode"=0, "Gradient Buffer"=2}, "Control"={"Sample Rate"=1, "PID gains"={"proportional gain (Kc)"=1.0, "integral time (Ti, min)"=0.01, "derivative time (Td, min)"=0.0}}, "Manual Temp Control"={"TargetTemp"=1.0, "Mode"=0, "Active"=FALSE}} ("Default values")) -> ("Data Acquisition.Camera.Calibration"=w342:T15)
        n154 = Bundle(cluster=w342, "Top Left"=w352, "Top Right"=w351, "Bottom Left"=w350, "Bottom Right"=w349, "Fixpoint"=w345, "Scan Area"=w348, "Fixpoint Area"=w344, "Well Pixels"=cluster{"X":i32, "Y":i32}[][] [], "Valid"=FALSE) -> (w353:T15)
        n155 = local read "Path"() -> (w341:path)
        n156 = Strip Path(path=w341) -> (stripped path=w337:path)  [unwired: 1 out]
        n157 = Strip Path(path=w337) -> (stripped path=w336:path)  [unwired: 1 out]
        n158 = call "CalibrationSavePrompt.vi"("Root Path"=w336) -> ("selected path"=w340:path, "cancel?"=w339:bool)
        n159 = case shown="False" w339 {
          tunnel: w354 -> [w361 w374]
          tunnel: [w360 w374] -> w338
          tunnel: w353 -> [w359 _]
          tunnel: w340 -> [w358 _]
          frame False {
            n160 = call <vilib>:"Check if File or Folder Exists.vi"("error in (no error)"=w361, "path"=w358) -> ("error out"=w365:errorcluster, "file or folder exists?"=w367:bool, "dup path"=w366:path)  [unwired: 7 in]
            n161 = case shown="False" w367 {
              tunnel: w366 -> [w368 w372]
              tunnel: w365 -> [w370 w373]
              tunnel: [w369 w373] -> w364
              tunnel: [w368 w372] -> w363
              frame False {
                n162 = Open/Create/Replace File(file path (use dialog)=w368, error in=w370, operation (0:open)=T10."create") -> (error out=w369:errorcluster)  [unwired: 3 in, 2 out]
              }
              frame True {
              }
            }
            n163 = Flatten To XML(6:w359) -> (2:w362:string)
            n164 = call-poly <vilib>:"Write to XML File.vi"("error in (no error)"=w364, "XML Input"=w362, "XML File Path"=w363) -> ("error out"=w360:errorcluster)  [unwired: 6 in, 2 out]
          }
          frame True {
          }
        }
        n165 = call <vilib>:"Add State(s) to Queue__JKI_lib_State_Machine.vi"("State(s) in (\"\")"=w357) -> ("States Out"=w356:string)  [unwired: 14 in]
      }
      frame "---------- UI ----------" {
        # "Do not put any code in this frame.\n(It is a separator no-op. You can make a copy of this frame to create a new UI frame)"
        n166 = call <vilib>:"Add State(s) to Queue__JKI_lib_State_Machine.vi"("State(s) in (\"\")"=w378) -> ("States Out"=w377:string)  [unwired: 14 in]
      }
      frame "UI: Initialize" {
        w379 = u32 0 items=["Grayscale", "Binary", "Gradient", "Rainbow", "Temperature", "User Defined", "Binary 16 Bit", "Gradient 16 Bit", "Rainbow 16 Bit", "Temperature 16 Bit", "User Defined 16 Bit"] ("Palette:Palette Type")
        w384 = T12 4 items=["Grayscale (U8)", "Grayscale (I16)", "Grayscale (SGL)", "Complex (CSG)", "RGB (U32)", "HSL (U32)", "RGB (U64)", "Grayscale (U16)"] ("Image Type")
        w392 = u32 1 items=["Zoom Tool"=8, "Selection Tool"=0, "Pan Tool"=9, "Point Tool"=1, "Line Tool"=2, "Rectangle Tool"=3, "Rotated Rectangle Tool"=12, "Polyline Tool"=10, "Polygon Tool"=5, "Freehand Tool"=11, "Closed Freehand Tool"=6, "Ellipse Tool"=4, "Annulus Tool"=7] ("Current ROI Tool")
        w393 = u32 15 items=["Default"=10, "Most Significant Bits"=11, "Full Dynamic"=12, "Downshift"=13, "Given Range"=14, "90% Dynamic"=15, "Given Percent Range"=16] ("16-bit Display Mapping:Conversion Method")
        # "Initialize the User Interface, here.\n(this is called automatically, by the Macro: Init)"
        n167 = call <vilib>:"Application Directory.vi"() -> ("Application Directory"=w388:path)
        n168 = Path To String(path=w388) -> (string=w390:string)
        n169 = call "IMAQ Create"("Image Name"="placeholder_img_TCC", "Image Type"=w384) -> ("New Image"=w387:T2)  [unwired: 3 in, 1 out]
        n170 = Concatenate Strings(w390, "\\camera_placeholder.png") -> (w389:string)
        n171 = String To Path(string=w389) -> (path=w391:path)
        n172 = call "IMAQ ReadFile 2"("Use File Path Image Type"=FALSE, "File Path"=w391, "Image"=w387) -> ("Image Out"=w382:T2)  [unwired: 4 in, 4 out]
        n173 = property on="Image" class="ImageControl"("16-bit Display Conversion Method"=w393) -> ()  [unwired: 2 in, 2 out]
        n174 = property on="Image" class="ImageControl"("Current ROI Tool"=w392, "Palette Type"=w379) -> ()  [unwired: 2 in, 2 out]
        n175 = local write "Display Mapping"(w393) -> ()
        n176 = local write "Image"(w382) -> ()
        n177 = local write "Path"(path "" ("Path")) -> ()
        n178 = property on="Image" class="ImageControl"("Zoom to Fit Mode"=TRUE) -> ()  [unwired: 2 in, 2 out]
        n179 = call <vilib>:"Add State(s) to Queue__JKI_lib_State_Machine.vi"("State(s) in Front (\"\")"="UI: Tutorial\n// UI: Progress >> Hide" ("State(s) in Front (\"\")"), "State(s) in (\"\")"=w398) -> ("States Out"=w397:string)  [unwired: 13 in]
      }
      frame "UI: Tutorial" {
        # "Initialize the User Interface, here.\n(this is called automatically, by the Macro: Init)"
        n180 = local read "State"() -> (w413:i32)
        n181 = case shown="2" w413 {
          tunnel: ["Load Calibration Image." "Select a Display Mapping that shows a clear image.\n\nSelect correct PCR size." w432 w450 w457 w464 "Select Well Radius so the center of each well is covered.\n\nGo to previous steps to adjust positions. Press done once satisfied."] -> w412
          tunnel: [_ _ _ _ _ _ w469] -> w411
          tunnel: [_ _ _ _ _ _ w469] -> w410
          tunnel: [_ w425 _ _ _ _ _] -> w409
          tunnel: [_ w425 _ _ _ _ _] -> w408
          tunnel: [w417 w425 w433 w447 w454 w461 _] -> w407
          tunnel: [_ w425 w439 w445 w451 w459 w469] -> w406
          tunnel: [TRUE _ _ _ _ _ _] -> w405
          tunnel: [_ _ w430 _ _ _ _] -> w404
          tunnel: w403 -> [_ _ w442 w448 w455 w462 _]
          tunnel: ["Step: 1/7" "Step: 2/7" "Step: 3/7" "Step: 4/7" "Step: 5/7" "Step: 6/7" "Step: 7/7"] -> w402
          tunnel: [_ _ _ _ _ _ w467] -> w401
          tunnel: [_ TRUE w439 w445 w451 w459 TRUE] -> w400
          tunnel: [_ 0 ("t") w436 3 ("t") 4 ("t") 5 ("t") 6 ("t")] -> w399
          frame 0, Default {
            n182 = local read "Path"() -> (w419:path)
            n183 = Empty String/Path?(string/path=w419) -> (empty?=w418:bool)
            n184 = Not(x=w418) -> (.not. x?=w417:bool)
          }
          frame 1 {
            w425 = TRUE
          }
          frame 2 {
            w439 = TRUE
            w443 = "Select Fix Point Cavity (Left Click) as shown (zoom with Mouse Wheel).\n\n"  # Select Fix Point Cavity (Left Click) as shown (zoom with Mouse Wheel).
            n185 = Unbundle By Name(w442) -> ("Points.Fixpoint.X"=w441:sgl)
            n186 = local read "Fixpoint Radius"() -> (w435:i32)
            n187 = Not Equal To 0?(x=w441) -> (x != 0?=w430:bool)
            n188 = Not Equal To 0?(x=w435) -> (x != 0?=w434:bool)
            n189 = And(x=w434, y=w430) -> (x .and. y?=w433:bool)
            n190 = Select(t="Set Fixpoint Radius so the cavity is appropriately filled as shown. ", s=w430, f="") -> (s? t:f=w431:string)
            n191 = Select(t=2, s=w430, f=1) -> (s? t:f=w436:i32)
            n192 = Concatenate Strings(w443, w431) -> (w432:string)
          }
          frame 3 {
            w445 = TRUE
            w450 = "Select Top Left corner of PCR plate as shown."  # Select Top Left corner of PCR plate as shown.
            n193 = Unbundle By Name(w448) -> ("Points.Top Left.X"=w449:sgl)
            n194 = Not Equal To 0?(x=w449) -> (x != 0?=w447:bool)
          }
          frame 4 {
            w451 = TRUE
            w457 = "Select Top Right corner of PCR plate as shown."  # Select Top Right corner of PCR plate as shown.
            n195 = Unbundle By Name(w455) -> ("Points.Top Right.X"=w456:sgl)
            n196 = Not Equal To 0?(x=w456) -> (x != 0?=w454:bool)
          }
          frame 5 {
            w459 = TRUE
            w464 = "Select Bottom Left corner of PCR plate as shown."  # Select Bottom Left corner of PCR plate as shown.
            n197 = Unbundle By Name(w462) -> ("Points.Bottom Left.X"=w463:sgl)
            n198 = Not Equal To 0?(x=w463) -> (x != 0?=w461:bool)
          }
          frame 6 {
            w469 = TRUE
            n199 = local read "Well Radius"() -> (w468:u32)
            n200 = Not Equal To 0?(x=w468) -> (x != 0?=w467:bool)
          }
        }
        "Tutorial" <- w412
        "Step" <- w402
        "Pict Ring" <- w399
        n201 = property on="Fixpoint Radius" class="DigNum (strict)"("Visible"=w404) -> ()  [unwired: 2 in, 2 out]
        n202 = property on="Path" class="Path"("Visible"=w405) -> ()  [unwired: 2 in, 2 out]
        n203 = property on="Well Radius" class="DigNum (strict)"("Visible"=w411) -> ()  [unwired: 2 in, 2 out]
        n204 = property on="Show All Points" class="Bool (strict)"("Visible"=w410) -> ()  [unwired: 2 in, 2 out]
        n205 = property on="Display Mapping" class="Ring (strict)"("Visible"=w409) -> ()  [unwired: 2 in, 2 out]
        n206 = property on="PCR Size" class="Ring (strict)"("Visible"=w408) -> ()  [unwired: 2 in, 2 out]
        n207 = property on="Next" class="Bool"("Visible"=w407) -> ()  [unwired: 2 in, 2 out]
        n208 = property on="Previous" class="Bool"("Visible"=w406) -> ()  [unwired: 2 in, 2 out]
        n209 = property on="Done" class="Bool"("Visible"=w401) -> ()  [unwired: 2 in, 2 out]
        n210 = property on="Pict Ring" class="Ring (strict)"("Visible"=w400) -> ()  [unwired: 2 in, 2 out]
        n211 = call <vilib>:"Add State(s) to Queue__JKI_lib_State_Machine.vi"("State(s) in (\"\")"=w416) -> ("States Out"=w415:string)  [unwired: 14 in]
      }
      frame "UI: Cursor Set" {
        # "Argument"
        # "Set and Unset Cursor Busy.\n(Usage: \"UI: Cursor Set >> Busy|Idle\")"
        n212 = case shown="\"Busy\"" w472 {
          tunnel: w474 -> [w479 w481]
          tunnel: [w478 w480] -> w473
          frame "Idle", Default {
            n213 = call <vilib>:"Unset Busy.vi"("error in (no error)"=w479) -> ("error out"=w478:errorcluster)  [unwired: 10 in]
          }
          frame "Busy" {
            n214 = call <vilib>:"Set Busy.vi"("error in (no error)"=w481) -> ("error out"=w480:errorcluster)  [unwired: 9 in, 1 out]
          }
        }
        n215 = call <vilib>:"Add State(s) to Queue__JKI_lib_State_Machine.vi"("State(s) in (\"\")"=w477) -> ("States Out"=w476:string)  [unwired: 14 in]
      }
      frame "UI: Front Panel State" {
        # "Argument"
        # "Set Front Panel Open or Closed\n(Usage: \"UI: Front Panel State >> Open|Close\")"
        n216 = Unbundle By Name(w484) -> ("Core.Current VI Reference"=w483:refnum<vi>)
        n217 = case shown="\"Close\", \"Closed\"" w482 {
          tunnel: w486 -> [w494 w509 w520 w533 w546]
          tunnel: [w496 w510 w522 w535 w548] -> w485
          tunnel: w483 -> [w495 w507 w521 w534 w547]
          frame "Open", "Standard", Default {
            w489 = T4."Standard" ("State")
            n218 = property class="VI"(reference=w495, error in=w494) -> (reference out=w492:refnum<vi>, error out=w493:errorcluster, "FP.State"=w491:T4)
            n219 = Not Equal?(x=w491, y=w489) -> (x != y?=w490:bool)
            n220 = case shown="True" w490 {
              tunnel: [w500 w502] -> w496
              tunnel: w493 -> [w499 w502]
              tunnel: w492 -> [w498 _]
              tunnel: w489 -> [w497 _]
              frame True {
                n221 = invoke class="VI" method="FP.Open"(reference=w498, error in=w499, "Activate"=TRUE, "State"=w497) -> (error out=w500:errorcluster)  [unwired: 1 in, 4 out]
              }
              frame False {
              }
            }
          }
          frame "Close", "Closed" {
            n222 = property class="VI"(reference=w507, error in=w509) -> (reference out=w506:refnum<vi>, error out=w508:errorcluster, "FP.State"=w504:T4)
            n223 = Not Equal?(x=w504, y=T4."Closed" ("Front Panel Window:State")) -> (x != y?=w503:bool)
            n224 = case shown="True" w503 {
              tunnel: [w511 w514] -> w510
              tunnel: w508 -> [w511 w513]
              tunnel: w506 -> [_ w512]
              frame False {
              }
              frame True {
                n225 = invoke class="VI" method="FP.Close"(reference=w512, error in=w513) -> (error out=w514:errorcluster)  [unwired: 1 in, 2 out]
              }
            }
          }
          frame "Hidden", "Hide" {
            w515 = T4."Hidden" ("State")
            n226 = property class="VI"(reference=w521, error in=w520) -> (reference out=w518:refnum<vi>, error out=w519:errorcluster, "FP.State"=w517:T4)
            n227 = Not Equal?(x=w517, y=w515) -> (x != y?=w516:bool)
            n228 = case shown="True" w516 {
              tunnel: [w526 w527] -> w522
              tunnel: w519 -> [w525 w527]
              tunnel: w518 -> [w524 _]
              tunnel: w515 -> [w523 _]
              frame True {
                n229 = invoke class="VI" method="FP.Open"(reference=w524, error in=w525, "State"=w523) -> (error out=w526:errorcluster)  [unwired: 2 in, 4 out]
              }
              frame False {
              }
            }
          }
          frame "Minimize", "Minimized" {
            w528 = T4."Minimized" ("State")
            n230 = property class="VI"(reference=w534, error in=w533) -> (reference out=w531:refnum<vi>, error out=w532:errorcluster, "FP.State"=w530:T4)
            n231 = Not Equal?(x=w530, y=w528) -> (x != y?=w529:bool)
            n232 = case shown="True" w529 {
              tunnel: [w539 w540] -> w535
              tunnel: w532 -> [w538 w540]
              tunnel: w531 -> [w537 _]
              tunnel: w528 -> [w536 _]
              frame True {
                n233 = invoke class="VI" method="FP.Open"(reference=w537, error in=w538, "State"=w536) -> (error out=w539:errorcluster)  [unwired: 2 in, 4 out]
              }
              frame False {
              }
            }
          }
          frame "Maximize", "Maximized" {
            w541 = T4."Maximized" ("State")
            n234 = property class="VI"(reference=w547, error in=w546) -> (reference out=w544:refnum<vi>, error out=w545:errorcluster, "FP.State"=w543:T4)
            n235 = Not Equal?(x=w543, y=w541) -> (x != y?=w542:bool)
            n236 = case shown="True" w542 {
              tunnel: [w552 w553] -> w548
              tunnel: w545 -> [w551 w553]
              tunnel: w544 -> [w550 _]
              tunnel: w541 -> [w549 _]
              frame True {
                n237 = invoke class="VI" method="FP.Open"(reference=w550, error in=w551, "State"=w549) -> (error out=w552:errorcluster)  [unwired: 2 in, 4 out]
              }
              frame False {
              }
            }
          }
        }
        n238 = call <vilib>:"Add State(s) to Queue__JKI_lib_State_Machine.vi"("State(s) in (\"\")"=w488) -> ("States Out"=w487:string)  [unwired: 14 in]
      }
      frame "---------- Macro ----------" {
        # "Do not put any code in this frame.\n(It is a separator no-op. You can make a copy of this frame to create a new Macro frame)"
        n239 = call <vilib>:"Add State(s) to Queue__JKI_lib_State_Machine.vi"("State(s) in (\"\")"=w557) -> ("States Out"=w556:string)  [unwired: 14 in]
      }
      frame "Macro: Initialize" {
        w558 = "// UI: Cursor Set >> Busy\nData: Initialize\nInitialize Core Data\nUI: Initialize\nUI: Front Panel State >> Show\nUI: Tutorial\nData: Load Image\n// Image: Draw\n// UI: Cursor Set >> Idle"  # // UI: Cursor Set >> Busy Data: Initialize Initialize Core Data UI: Initialize UI: Front Panel State >> Show UI: Tutorial Data: Load Image // Image: Draw // UI: Cursor Set >> Idle
        # "Initialization Macro\n(This is called once, when the VI starts)"
        n240 = call <vilib>:"Add State(s) to Queue__JKI_lib_State_Machine.vi"("State(s) in Front (\"\")"=w558, "State(s) in (\"\")"=w562) -> ("States Out"=w561:string)  [unwired: 13 in]
      }
      frame "Macro: Exit" {
        # "Exit Macro\n(This is called once, when the VI exits)"
        n241 = Unbundle By Name(w570) -> ("Core.Close Panel on Exit?"=w569:bool)
        n242 = Select(t="UI: Front Panel State >> Close", s=w569, f="") -> (s? t:f=w566:string)
        n243 = call <vilib>:"Add State(s) to Queue__JKI_lib_State_Machine.vi"("State(s) in Front (\"\")"="Data: Cleanup" ("State(s) in Front (\"\")"), "State(s) in (\"\")"=w566, "State(s) at Back (\"\")"="Exit") -> ("States Out"=w564:string)  [unwired: 12 in]
        n244 = call <vilib>:"Add State(s) to Queue__JKI_lib_State_Machine.vi"("State(s) in Front (\"\")"=w564, "State(s) in (\"\")"=w573) -> ("States Out"=w572:string)  [unwired: 13 in]
      }
      frame "---------- Image ----------" {
        # "Template Separator\n(You can make a copy of, or modify, this frame)"
        n245 = call <vilib>:"Add State(s) to Queue__JKI_lib_State_Machine.vi"("State(s) in (\"\")"=w577) -> ("States Out"=w576:string)  [unwired: 14 in]
      }
      frame "Image: Draw" {
        # "Template Separator\n(You can make a copy of, or modify, this frame)"
        n246 = call <vilib>:"Add State(s) to Queue__JKI_lib_State_Machine.vi"("State(s) in Front (\"\")"="UI: Cursor Set >> Busy\nImage: Clear ROI\nImage: Set ROI\nImage: Draw Fixedpoint\nImage: Calculate BR\nImage: Calculate y space\nImage: Calculate x space\nImage: Calculate Positions\nImage: Drawlines\nImage: Draw Points\nUI: Cursor Set >> Idle" ("State(s) in Front (\"\")"), "State(s) in (\"\")"=w582) -> ("States Out"=w581:string)  [unwired: 13 in]
      }
      frame "Image: Redraw" {
        # "Template Separator\n(You can make a copy of, or modify, this frame)"
        n247 = call <vilib>:"Add State(s) to Queue__JKI_lib_State_Machine.vi"("State(s) in Front (\"\")"="UI: Cursor Set >> Busy\nImage: Clear ROI\nImage: Drawlines\nImage: Draw Points\nImage: Calculate Temps\nUI: Cursor Set >> Idle" ("State(s) in Front (\"\")"), "State(s) in (\"\")"=w587) -> ("States Out"=w586:string)  [unwired: 13 in]
      }
      frame "Image: Drawlines" {
        # "Template Separator\n(You can make a copy of, or modify, this frame)"
        n248 = Unbundle By Name(w588) -> ("Points.Top Left.X"=w604:sgl, "Points.Top Right.X"=w603:sgl, "Points.Bottom Left.X"=w602:sgl, "Points.Bottom Right.X"=w601:sgl)
        n249 = Equal To 0?(x=w601) -> (x = 0?=w591:bool)
        n250 = Equal To 0?(x=w602) -> (x = 0?=w590:bool)
        n251 = Or(x=w590, y=w591) -> (x .or. y?=w589:bool)
        n252 = Equal To 0?(x=w604) -> (x = 0?=w600:bool)
        n253 = Equal To 0?(x=w603) -> (x = 0?=w599:bool)
        n254 = Select(t="", s=w590, f="Image: Draw Line >> TL_BL\n") -> (s? t:f=w596:string)
        n255 = Select(t="", s=w589, f="Image: Draw Line >> TR_BR\nImage: Draw Line >> BL_BR\nImage: Draw Line >> Vertical\nImage: Draw Line >> Horizontal") -> (s? t:f=w593:string)
        n256 = case shown="False" w600 {
          tunnel: w599 -> [w611 _]
          tunnel: w596 -> [w610 _]
          tunnel: w593 -> [w609 _]
          tunnel: [w608 _] -> w592
          frame False {
            n257 = case shown="False" w611 {
              tunnel: w610 -> [w614 _]
              tunnel: w609 -> [w613 _]
              tunnel: [w612 _] -> w608
              frame False {
                n258 = Concatenate Strings("Image: Draw Line >> TL_TR\n", w614, w613) -> (w612:string)
              }
              frame True {
              }
            }
          }
          frame True {
          }
        }
        n259 = call <vilib>:"Add State(s) to Queue__JKI_lib_State_Machine.vi"("State(s) in Front (\"\")"=w592, "State(s) in (\"\")"=w607) -> ("States Out"=w606:string)  [unwired: 13 in]
      }
      frame "Image: Draw Fixedpoint" {
        # "Template Separator\n(You can make a copy of, or modify, this frame)"
        n260 = Unbundle By Name(w622) -> ("Image Out"=w619:T2, "Points.Fixpoint"=w621:T3)
        n261 = Build Array(w621) -> (w620:T3[])
        n262 = call "TCam_CenterArray.vi"("Size"="Fixpoint Radius", "Point Array"=w620, "Image in"=w619) -> ("Image"=w618:T2)  [unwired: 3 in, 1 out]
        n263 = local write "Image"(w618) -> ()
        n264 = call <vilib>:"Add State(s) to Queue__JKI_lib_State_Machine.vi"("State(s) in (\"\")"=w624) -> ("States Out"=w623:string)  [unwired: 14 in]
      }
      frame "Image: Clear ROI" {
        # "Your code here.\n(You can make a copy of, or modify, this frame)"
        n265 = Unbundle By Name(w628) -> ("Image Out"=w627:T2)
        n266 = call "IMAQ Clear Overlay"("error in (no error)"=w626, "Image"=w627) -> ("error out"=w625:errorcluster)  [unwired: 8 in, 1 out]
        n267 = call <vilib>:"Add State(s) to Queue__JKI_lib_State_Machine.vi"("State(s) in (\"\")"=w630) -> ("States Out"=w629:string)  [unwired: 14 in]
      }
      frame "Image: Calculate x space" {
        # "Your code here.\n(You can make a copy of, or modify, this frame)"
        n268 = Unbundle By Name(w639) -> ("Points.Top Left"=w645:T3, "Points.Top Right"=w644:T3)
        n269 = case shown="1" "PCR Size" {
          tunnel: [24 12] -> w631
          frame 0, Default {
          }
          frame 1 {
          }
        }
        n270 = Unbundle(w644) -> ("X"=w643:sgl, "Y"=w641:sgl)
        n271 = Unbundle(w645) -> ("X"=w642:sgl, "Y"=w640:sgl)
        n272 = Subtract(x=w643, y=w642) -> (x-y=w636:sgl)
        n273 = Decrement(x=w631) -> (x-1=w635:i32)
        n274 = Subtract(x=w641, y=w640) -> (x-y=w634:sgl)
        n275 = Divide(x=w636, y=w635) -> (x/y=w637:sgl)
        n276 = Divide(x=w634, y=w635) -> (x/y=w633:sgl)
        n277 = Bundle By Name(cluster=w639, "Points.x_space"=w637, "Points.y_space"=w633) -> (w638:T1)
        n278 = call <vilib>:"Add State(s) to Queue__JKI_lib_State_Machine.vi"("State(s) in (\"\")"=w648) -> ("States Out"=w647:string)  [unwired: 14 in]
      }
      frame "Image: Calculate BR" {
        # "Your code here.\n(You can make a copy of, or modify, this frame)"
        n279 = Unbundle By Name(w659) -> ("Points.Top Left"=w665:T3, "Points.Top Right"=w664:T3, "Points.Bottom Left"=w657:T3)
        n280 = Unbundle(w665) -> ("X"=w662:sgl, "Y"=w660:sgl)
        n281 = Unbundle(w664) -> ("X"=w663:sgl, "Y"=w661:sgl)
        n282 = Unbundle(w657) -> ("X"=w656:sgl, "Y"=w654:sgl)
        n283 = Subtract(x=w663, y=w662) -> (x-y=w655:sgl)
        n284 = Subtract(x=w661, y=w660) -> (x-y=w653:sgl)
        n285 = Add(x=w656, y=w655) -> (x+y=w651:sgl)
        n286 = Add(x=w653, y=w654) -> (x+y=w652:sgl)
        n287 = Bundle By Name(cluster=w659, "Points.Bottom Right.X"=w651, "Points.Bottom Right.Y"=w652) -> (w658:T1)
        n288 = call <vilib>:"Add State(s) to Queue__JKI_lib_State_Machine.vi"("State(s) in (\"\")"=w668) -> ("States Out"=w667:string)  [unwired: 14 in]
      }
      frame "Image: Calculate y space" {
        # "Your code here.\n(You can make a copy of, or modify, this frame)"
        n289 = local read "PCR Size"() -> (w670:u16)
        n290 = Unbundle By Name(w677) -> ("Points.Top Left"=w683:T3, "Points.Bottom Left"=w682:T3)
        n291 = case shown="1" w670 {
          tunnel: [16 8] -> w669
          frame 0, Default {
          }
          frame 1 {
          }
        }
        n292 = Unbundle(w682) -> ("X"=w681:sgl, "Y"=w679:sgl)
        n293 = Unbundle(w683) -> ("X"=w680:sgl, "Y"=w678:sgl)
        n294 = Subtract(x=w681, y=w680) -> (x-y=w674:sgl)
        n295 = Decrement(x=w669) -> (x-1=w673:i32)
        n296 = Subtract(x=w679, y=w678) -> (x-y=w672:sgl)
        n297 = Divide(x=w674, y=w673) -> (x/y=w675:sgl)
        n298 = Divide(x=w672, y=w673) -> (x/y=w671:sgl)
        n299 = Bundle By Name(cluster=w677, "Points.x space 2"=w675, "Points.y space 2"=w671) -> (w676:T1)
        n300 = call <vilib>:"Add State(s) to Queue__JKI_lib_State_Machine.vi"("State(s) in (\"\")"=w686) -> ("States Out"=w685:string)  [unwired: 14 in]
      }
      frame "Image: Set ROI" {
        # "Your code here.\n(You can make a copy of, or modify, this frame)"
        n301 = Unbundle By Name(w695) -> ("State"=w693:i32)
        n302 = case shown="2..5" w693 {
          tunnel: w693 -> [_ w707]
          tunnel: w695 -> [_ w705]
          tunnel: w694 -> [w700 w704]
          tunnel: [w700 w703] -> w692
          tunnel: [T11 {"Global Rectangle"=[], "Contours"=[]} ("ROI Descriptor") w702] -> w691
          tunnel: [w698 w701] -> w689
          frame 0, Default {
            w698 = u32 0 items=["Zoom Tool"=8, "Selection Tool"=0, "Pan Tool"=9, "Point Tool"=1, "Line Tool"=2, "Rectangle Tool"=3, "Rotated Rectangle Tool"=12, "Polyline Tool"=10, "Polygon Tool"=5, "Freehand Tool"=11, "Closed Freehand Tool"=6, "Ellipse Tool"=4, "Annulus Tool"=7] ("Current ROI Tool")
          }
          frame 2..5 {
            w701 = u32 1 items=["Zoom Tool"=8, "Selection Tool"=0, "Pan Tool"=9, "Point Tool"=1, "Line Tool"=2, "Rectangle Tool"=3, "Rotated Rectangle Tool"=12, "Polyline Tool"=10, "Polygon Tool"=5, "Freehand Tool"=11, "Closed Freehand Tool"=6, "Ellipse Tool"=4, "Annulus Tool"=7] ("Current ROI Tool")
            n303 = case shown="5" w707 {
              tunnel: [w709 w711 w713 w715] -> w706
              tunnel: w705 -> [w708 w710 w712 w714]
              frame 2, Default {
                n304 = Unbundle By Name(w708) -> ("Points.Fixpoint"=w709:T3)
              }
              frame 3 {
                n305 = Unbundle By Name(w710) -> ("Points.Top Left"=w711:T3)
              }
              frame 4 {
                n306 = Unbundle By Name(w712) -> ("Points.Top Right"=w713:T3)
              }
              frame 5 {
                n307 = Unbundle By Name(w714) -> ("Points.Bottom Left"=w715:T3)
              }
            }
            n308 = call "IMAQ Convert Point to ROI"("error in (no error)"=w704, "Point"=w706) -> ("error out"=w703:errorcluster, "ROI Descriptor"=w702:T11)  [unwired: 7 in]
          }
        }
        n309 = property on="Image" class="ImageControl"("Current ROI Tool"=w689) -> ()  [unwired: 2 in, 2 out]
        n310 = property on="Image" class="ImageControl"(error in=w692, "ROI"=w691) -> (error out=w690:errorcluster)  [unwired: 1 in, 1 out]
        n311 = call <vilib>:"Add State(s) to Queue__JKI_lib_State_Machine.vi"("State(s) in (\"\")"=w697) -> ("States Out"=w696:string)  [unwired: 14 in]
      }
      frame "Image: Draw Line" {
        w716 = u32 1  # Width_Minor
        w717 = u32 2  # Width
        # "Your code here.\n(You can make a copy of, or modify, this frame)"
        n312 = Unbundle By Name(w721) -> ("Image Out"=w722:T2)
        n313 = case shown="\"Vertical\"" w723 {
          tunnel: w722 -> [w727 w735 w744 w751 w757 w762 w771]
          tunnel: w721 -> [_ w736 w745 w747 w753 w766 w775]
          tunnel: [w727 w730 w743 w750 w756 w758 w767] -> w720
          tunnel: w719 -> [w726 w734 w742 w749 w755 w760 w770]
          tunnel: [w726 w729 w741 w748 w754 w759 w769] -> w718
          tunnel: w717 -> [_ w728 w737 _ _ w761 w768]
          tunnel: w716 -> [_ _ _ w746 w752 _ _]
          frame "False", Default {
          }
          frame "TL_TR" {
            n314 = Unbundle By Name(w736) -> ("Points.Top Left"=w733:T3, "Points.Top Right"=w732:T3)
            n315 = Build Array(w733, w732) -> (w731:T3[])
            n316 = call "IMAQ Overlay Multiple Lines 2"("Image"=w735, "Line End Points"=w731, "error in (no error)"=w734, "Width"=w728) -> ("Image Out"=w730:T2, "error out"=w729:errorcluster)  [unwired: 10 in]
          }
          frame "TL_BL" {
            n317 = Unbundle By Name(w745) -> ("Points.Top Left"=w740:T3, "Points.Bottom Left"=w739:T3)
            n318 = Build Array(w740, w739) -> (w738:T3[])
            n319 = call "IMAQ Overlay Multiple Lines 2"("Image"=w744, "Line End Points"=w738, "error in (no error)"=w742, "Width"=w737) -> ("Image Out"=w743:T2, "error out"=w741:errorcluster)  [unwired: 10 in]
          }
          frame "Vertical" {
            n320 = call "TCam_VerticalLines.vi"("Width"=w746, "error in (no error)"=w749, "Cluster"=w747, "Refnum in"=w751) -> ("error out"=w748:errorcluster, "Refnum out"=w750:T2)  [unwired: 6 in]
          }
          frame "Horizontal" {
            n321 = call "TCam_HorizontalLines.vi"("Width"=w752, "error in (no error)"=w755, "Cluster"=w753, "Refnum in"=w757) -> ("error out"=w754:errorcluster, "Refnum out"=w756:T2)  [unwired: 6 in]
          }
          frame "TR_BR" {
            n322 = Unbundle By Name(w766) -> ("Points.Top Right"=w765:T3, "Points.Bottom Right"=w764:T3)
            n323 = Build Array(w765, w764) -> (w763:T3[])
            n324 = call "IMAQ Overlay Multiple Lines 2"("Image"=w762, "Line End Points"=w763, "error in (no error)"=w760, "Width"=w761) -> ("Image Out"=w758:T2, "error out"=w759:errorcluster)  [unwired: 10 in]
          }
          frame "BL_BR" {
            n325 = Unbundle By Name(w775) -> ("Points.Bottom Left"=w774:T3, "Points.Bottom Right"=w773:T3)
            n326 = Build Array(w774, w773) -> (w772:T3[])
            n327 = call "IMAQ Overlay Multiple Lines 2"("Image"=w771, "Line End Points"=w772, "error in (no error)"=w770, "Width"=w768) -> ("Image Out"=w767:T2, "error out"=w769:errorcluster)  [unwired: 10 in]
          }
        }
        n328 = local write "Image"(w720) -> ()
        n329 = call <vilib>:"Add State(s) to Queue__JKI_lib_State_Machine.vi"("State(s) in (\"\")"=w725) -> ("States Out"=w724:string)  [unwired: 14 in]
      }
      frame "Image: Draw Points" {
        # "Your code here.\n(You can make a copy of, or modify, this frame)"
        n330 = Unbundle By Name(w777) -> ("Points.Top Left.X"=w786:sgl, "Points.Top Right.X"=w785:sgl, "Points.Bottom Left.X"=w784:sgl, "Points.Bottom Right.X"=w783:sgl)
        n331 = Equal To 0?(x=w786) -> (x = 0?=w782:bool)
        n332 = Equal To 0?(x=w785) -> (x = 0?=w781:bool)
        n333 = Equal To 0?(x=w784) -> (x = 0?=w780:bool)
        n334 = Equal To 0?(x=w783) -> (x = 0?=w779:bool)
        n335 = Unbundle By Name(w777) -> ("Image Out"=w788:T2)
        n336 = Compound Arithmetic op=OR(w782, w781, w780, w779) -> (w778:bool)
        n337 = case shown="False" w778 {
          tunnel: w788 -> [w798 _]
          tunnel: w777 -> [w793 w799]
          tunnel: [w791 w799] -> w776
          frame False {
            n338 = local read "Points"() -> (w797:T3[])
            n339 = call "TCam_CenterArray.vi"("draw all?"="Show All Points", "Size"="Well Radius", "Point Array"=w797, "Image in"=w798) -> ("Array"=w792:cluster{"X":i32, "Y":i32}[][], "Image"=w795:T2)  [unwired: 2 in]
            n340 = local write "Image"(w795) -> ()
            n341 = Bundle By Name(cluster=w793, "Points.Pixels"=w792) -> (w791:T1)
          }
          frame True {
          }
        }
        n342 = call <vilib>:"Add State(s) to Queue__JKI_lib_State_Machine.vi"("State(s) in (\"\")"=w790) -> ("States Out"=w789:string)  [unwired: 14 in]
      }
      frame "Image: Calculate Positions" {
        # "Your code here.\n(You can make a copy of, or modify, this frame)"
        n343 = Unbundle By Name(w801) -> ("Points.Top Left.X"=w809:sgl, "Points.Top Right.X"=w808:sgl, "Points.Bottom Left.X"=w807:sgl, "Points.Bottom Right.X"=w806:sgl)
        n344 = Equal To 0?(x=w809) -> (x = 0?=w805:bool)
        n345 = Equal To 0?(x=w808) -> (x = 0?=w804:bool)
        n346 = Equal To 0?(x=w807) -> (x = 0?=w803:bool)
        n347 = Equal To 0?(x=w806) -> (x = 0?=w802:bool)
        n348 = Compound Arithmetic op=OR(w805, w804, w803, w802) -> (w800:bool)
        n349 = case shown="False" w800 {
          tunnel: w801 -> [w813 _]
          frame False {
            n350 = local read "PCR Size"() -> (w814:u16)
            n351 = call "TCam_PointCalculator.vi"("Cluster"=w813, "Size"=w814) -> ("Points"=→"Points":T3[])  [unwired: 9 in]
          }
          frame True {
          }
        }
        n352 = call <vilib>:"Add State(s) to Queue__JKI_lib_State_Machine.vi"("State(s) in (\"\")"=w812) -> ("States Out"=w811:string)  [unwired: 14 in]
      }
    }
  }
  "State out" <- "Data: Load Thermal Calibration"
